vi "Lockin_sweep.vi"(0 "Transport":refnum<class "Transport.lvclass">, 3 "error in (no error)":errorcluster) -> (7 "Transport out":refnum<class "Transport.lvclass">, 10 "error out":errorcluster)   [LabVIEW 2019, in "Transport.lvclass"]
doc: "This VI uses the Lockin Sweep Method. That is, you tell the lockin to sweep from Start to End in a certain amount of time. The lockin will run independently while it executes the sweep. While the lockin is sweeping, this VI will poll the lockin once per second to get a snapshot of current results and the sweep status (sweeping or not sweeping). When the lockin is finished sweeping this VI will ask for the final sweep results and save them. The spacing between points is determined by the \"Fs Output\" control in the Lockin."
uses:
  Transport.lvclass
  <userlib>/LevyLab/Lockin-Multichannel/Instrument.DAQ/Typedefs/Sweep.Channel--Cluster--Array.ctl
  <userlib>/LevyLab/Lockin-Multichannel/Instrument.DAQ/Typedefs/Sweep.Channel--Cluster.ctl
  <userlib>/LevyLab/Lockin-Multichannel/Instrument.DAQ/Typedefs/Sweep.Pattern--Enum.ctl
  Transport.lvclass/Transport.ctl
  Control Experiment/Control Experiment.lvclass/Control Experiment.ctl
  Control Experiment/Typedefs/Instrument Types--enum.ctl
  <userlib>/LevyLab/Lockin-Multichannel/Instrument.Lockin/Typedefs/Results Type--Enum.ctl
  <userlib>/LevyLab/Lockin-Multichannel/Instrument.DAQ/Typedefs/Sweep.Configuration--Cluster.ctl
  <userlib>/LevyLab/Instrument Framework/Instrument Types/Cryostat/Typedefs/Magnet Axis--Enum.ctl
  Typedefs/Lockin_Sweep JSON--Cluster.ctl
  d7da78e6-7697-4005-8475-e4e7ed229128.vi
  <vilib>/PRIrvin/XY Utilities/subVIs/Multiply float (multiple).vi
  <vilib>/PRIrvin/XY Utilities/subVIs/Divide float (multiple).vi
  ac72d6f7-f5c3-431a-8621-5120436d0f52.vi
  217905a9-ad64-4e54-8703-31da4ffbd4c0.vi
  9896b5e5-a649-4b1b-acc0-fd49b17a1bc1.vi
  ac72d6f7-f5c3-431a-8621-5120436d0f52.vi/7eee748f-304e-47d8-aeea-bfc744331f26.vi
  ac72d6f7-f5c3-431a-8621-5120436d0f52.vi/d9440ba2-8dc0-48fa-8208-7fa22d71755a.vi
  <userlib>/LevyLab/Instrument Framework/Instrument/Instrument.lvclass
  C:/Program Files/National Instruments/LabVIEW 2019/vi.lib/JKI/JKI SMO/SMO/SMO.lvclass
  <userlib>/LevyLab/Instrument Framework/Instrument Types/Cryostat/Instrument.Cryostat.lvclass
  <userlib>/LevyLab/Lockin-Multichannel/Instrument.Lockin/Instrument.Lockin.lvclass
  C:/Program Files/National Instruments/LabVIEW 2019/user.lib/LevyLab/Instrument Framework/Instrument Types/Lockin/Instrument.LockinAPI.lvclass
  <userlib>/LevyLab/Debug/Debug/Get Debug Mode.vi
  <userlib>/LevyLab/Lockin-Multichannel/Instrument.Lockin/Private/Lockin.Remote Client.vi
  <vilib>/JDP Science/JSONtext/Variant to JSON Text.vi
  Control Experiment/subVIs/String Label.vi
  <vilib>/JKI/JKI SMO/SMO/SMO.lvclass
  Control Experiment/Control Experiment.lvclass
  <vilib>/JDP Science/JSONtext/LVClass Serializer/JSONtext LVClass Serializer.lvclass
  <userlib>/LevyLab/Instrument Framework/Instrument Types/CBridge/Instrument.CBridge.lvclass
  <userlib>/LevyLab/Instrument Framework/Instrument Types/Strain/Instrument.Strain.lvclass
  <userlib>/LevyLab/Instrument Framework/Instrument Types/Delay Line/Instrument.DelayLine.lvclass
  <userlib>/LevyLab/Lockin-Multichannel/Instrument.DAQ/Instrument.DAQ.lvclass
  <vilib>/PRIrvin/XY Utilities/xy_utilities.lvlib
  <vilib>/Utility/Data Type/NI_Data Type.lvlib
  <userlib>/LevyLab/Instrument Framework/Instrument Types/Lockin/Instrument.LockinAPI.lvclass
  <userlib>/LevyLab/Instrument Framework/Instrument Types/Amplifier/Instrument.Amplifier.lvclass
  <userlib>/LevyLab/Instrument Framework/Instrument Types/VNA/Instrument.VNA.lvclass
  <userlib>/LevyLab/Instrument Framework/Instrument Types/VSource/Instrument.VSource.lvclass
  Attributes/Instrument Attributes.lvlib
  <userlib>/LevyLab/Debug/Debug.lvlib
panel:
  in  "Start":bool
  in  "stop":bool
  out "Tab Control":T1(tab)
  in  "refresh (ms)":u32=1000
  out "state history":string
  in  "Sweep Tables":cluster{"Ch":i32, "Table":dbl[]}[](array[cluster]) {"Table" format="%#_3p"; "Ch" min=1 max=16}
  in  "Emergency Stop Visible?":bool
  out "elapsed time (s)":i32=231
  out "Experiment Comments":string
  out "Experiment Folder":string
  out "time b/w points (ms)":u32=1037
  in  "Sweep Channels":T2 {"Table" format="%#_1f"; "Channel" min=1 max=128; "Start" format="%#_6p"; "End" format="%#_6p"}
  in  "Sweep Time (s)":dbl
  in  "Initial Wait (s)":dbl
  in  "Return to Start":bool
  out "Instrument Status":string
  in  "Emergency Stop 1":bool caption="Emergency Stop"
  out "Lockin (X)":cluster{"Wavenumber":dbl[], "Data":dbl[]}[](graph)
  out "Lockin (Y)":cluster{"Wavenumber":dbl[], "Data":dbl[]}[](graph)
  in  "Units":enum16{"ohms & siemens", "h/e2 & e2/h"}(ring)
  out "Resistance":cluster{"X-array":dbl[], "Y-array":dbl[]}[](graph)
  out "Conductance":cluster{"X-array":dbl[], "Y-array":dbl[]}[](graph)
  in  "Emergency Stop 2":bool caption="Emergency Stop"
  out "AI":cluster{"Wavenumber":dbl[], "Data":dbl[]}[](graph)
  out "AO":cluster{"Wavenumber":dbl[], "Data":dbl[]}[](graph)
  in  "Emergency Stop 3":bool caption="Emergency Stop"
  out "2 Terminal":cluster{"Wavenumber":dbl[], "Data":dbl[]}[](graph)
  out "4 Terminal":cluster{"Wavenumber":dbl[], "Data":dbl[]}[](graph)
  in  "Emergency Stop 4":bool caption="Emergency Stop"
  # "Configuration"
  # "Status"
  # "Metadata*"
  # "VI Description"
  # "Run a sweep on the lockin itself. The lockin is told to sweep from Start to End over a set time, and it runs the sweep on its own. While it sweeps, this VI polls the lockin once per fresh time for a snapshot of the current results and the sweep status. When the sweep finishes, it reads the final sweep results and saves them. The point spacing is set by the lockin's \"Fs Output\" control."
  # "*Change these values in Transport Server"
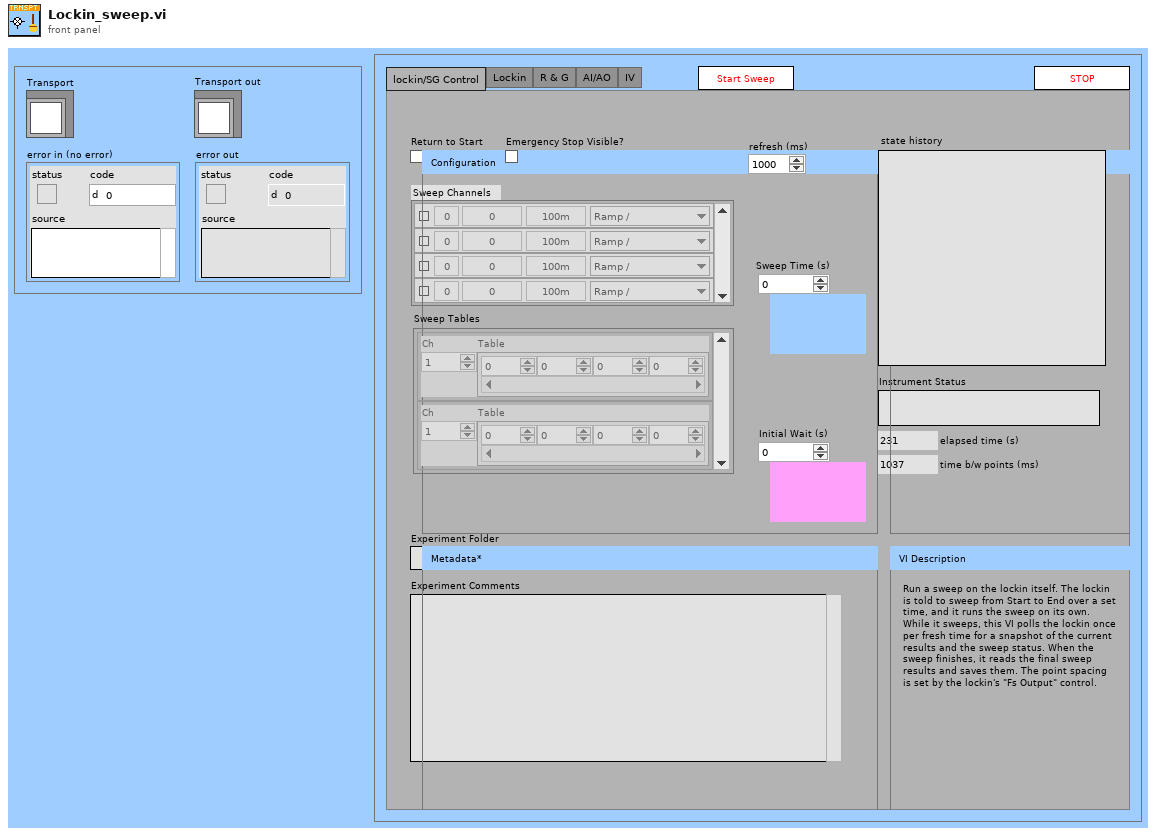
[diagram p1: front panel]
types:
  T1 = enum32{"lockin/SG Control", "Lockin", "R & G", "AI/AO", "IV"}
  T2 = typedef "Instrument.Lockin.lvlib/Instrument.DAQ.lvclass/Sweep.Channel--Cluster--Array.ctl" = T3[]
  T3 = typedef "Instrument.Lockin.lvlib/Instrument.DAQ.lvclass/Sweep.Channel--Cluster.ctl" = cluster{"Enable?":bool, "Channel":u16, "Start":dbl, "End":dbl, "Pattern":T4, "Table":dbl[]}
  T4 = typedef "Instrument.Lockin.lvlib/Instrument.DAQ.lvclass/Sweep.Pattern--Enum.ctl" = enum16{"Ramp /", "Ramp /\\", "Smooth Ramp _/", "Smooth Ramp _/\\_", "Table"}
  T5 = enum32{"Invalid", "Standard", "Closed", "Hidden", "Minimized", "Maximized"}
  T6 = enum32{"invalid app kind", "Development System", "Run Time System", "Student Edition", "Embedded LabVIEW", "Evaluation", "Custom"}
  T7 = enum32{"Bad", "Idle", "Run top level", "Running"}
  T8 = typedef "Control Experiment.lvclass/Instrument Types--enum.ctl" = enum16{"DAQ", "Amplifier", "Temperature", "Magnet", "Rotator", "Level", "Capacitance", "Delay Line", "Strain Cell", "VNA", "Source"}
  T9 = typedef "Instrument.Lockin.lvlib/Instrument.Lockin.lvclass/Results Type--Enum.ctl" = enum16{"X", "Y", "R", "Theta", "Mean"}
  T10 = typedef "Instrument.Lockin.lvlib/Instrument.DAQ.lvclass/Sweep.Configuration--Cluster.ctl" = cluster{"sweepTime":dbl, "initialWaitTime":dbl, "returnToStart":bool, "sweepChannels":T2}
  T11 = typedef "Instrument.Cryostat.lvclass/Magnet Axis--Enum.ctl" = enum16{"X", "Y", "Z"}
  T12 = typedef "Transport.lvclass/Lockin_Sweep JSON--Cluster.ctl" = cluster{"initialWaitTime":dbl, "sweepTime":dbl, "Return to Start":bool, "sweepChannels":T2, "sweepTables":cluster{"Ch":i32, "Table":dbl[]}[]}
  T13 = typedef "Control Experiment.lvclass/Instrument Classes--cluster.ctl" = cluster{"DAQ":refnum<class "Instrument.LockinAPI.lvclass">, "Amplifier":refnum<class "Instrument.Amplifier.lvclass">, "Temperature":refnum<class "Instrument.Cryostat.lvclass">, "Magnet":refnum<class "Instrument.Cryostat.lvclass">, "Rotator":refnum<class "Instrument.Cryostat.lvclass">, "Level":refnum<class "Instrument.Cryostat.lvclass">, "Capacitance":refnum<class "Instrument.CBridge.lvclass">, "Delay Line":refnum<class "Instrument.DelayLine.lvclass">, "Strain Cell":refnum<class "Instrument.Strain.lvclass">, "VNA":refnum<class "Instrument.VNA.lvclass">, "Source":refnum<class "Instrument.VSource.lvclass">}
  T14 = cluster{"Core":cluster{"Current VI Reference":refnum<vi>, "Close Panel on Exit?":bool}, "Transport":refnum<class "Transport.lvclass">, "C.E.":refnum<class "Control Experiment.lvclass">, "Instruments":T13, "Time":dbl, "Temperature":dbl, "Magnet":dbl, "Results (Dictionary)":cluster{"key":string, "value":dbl}[], "Sweep Value":dbl, "ms [0]":u32, "ms [i]":u32, "Execution:State":enum32{"Bad", "Idle", "Run top level", "Running"}, "Run Time System?":bool, "AO Waveforrm":waveform(dbl)[], "AI Waveform":waveform(dbl)[], "Sweep_AO":waveform(dbl)[], "Sweep_AI":waveform(dbl)[], "Sweep_X":waveform(dbl)[], "Sweep_Y":waveform(dbl)[], "Amplitude":dbl[], "UI stop":bool}
  T15 = cluster{"Current VI Reference":refnum<vi>, "Close Panel on Exit?":bool}
  T16 = cluster{"I-":i32, "I+":i32, "V1-":i32, "V1+":i32, "I2-":i32, "I2+":i32, "V2-":i32, "V2+":i32}
  T17 = typedef "Instrument.LockinAPI.lvclass/LockinAPI.getState.states--enum.ctl" = enum16{"idle", "created", "started", "stopped", "sweeping"}
  T18 = typedef "Instrument.Lockin.lvlib/Instrument.DAQ.lvclass/AO.Channel--Cluster--Array.ctl" = T19[]
  T19 = typedef "Instrument.Lockin.lvlib/Instrument.DAQ.lvclass/AO.Channel--Cluster.ctl" = cluster{"Enable?":bool, "Channel":i32, "Amplitude":dbl, "Offset":dbl, "Frequency":dbl, "Phase":dbl, "Function":T20, "Sweeping?":bool, "Limit AC":bool, "Limit DC?":bool, "Duty Cycle":bool}
  T20 = typedef "Instrument.Lockin.lvlib/Instrument.DAQ.lvclass/AO.Channel.Function--Enum.ctl" = enum16{"sine", "square", "triangle", "saw"}
  T21 = typedef "Instrument.LockinAPI.lvclass/LockinAPI.SweepData--Cluster.ctl" = cluster{"AO":waveform(dbl)[], "AI":waveform(dbl)[], "X":waveform(dbl)[], "Y":waveform(dbl)[]}
  T22 = typedef "LV-Data.lvclass/Dictionary--cluster.ctl" = cluster{"key":string, "value":variant}
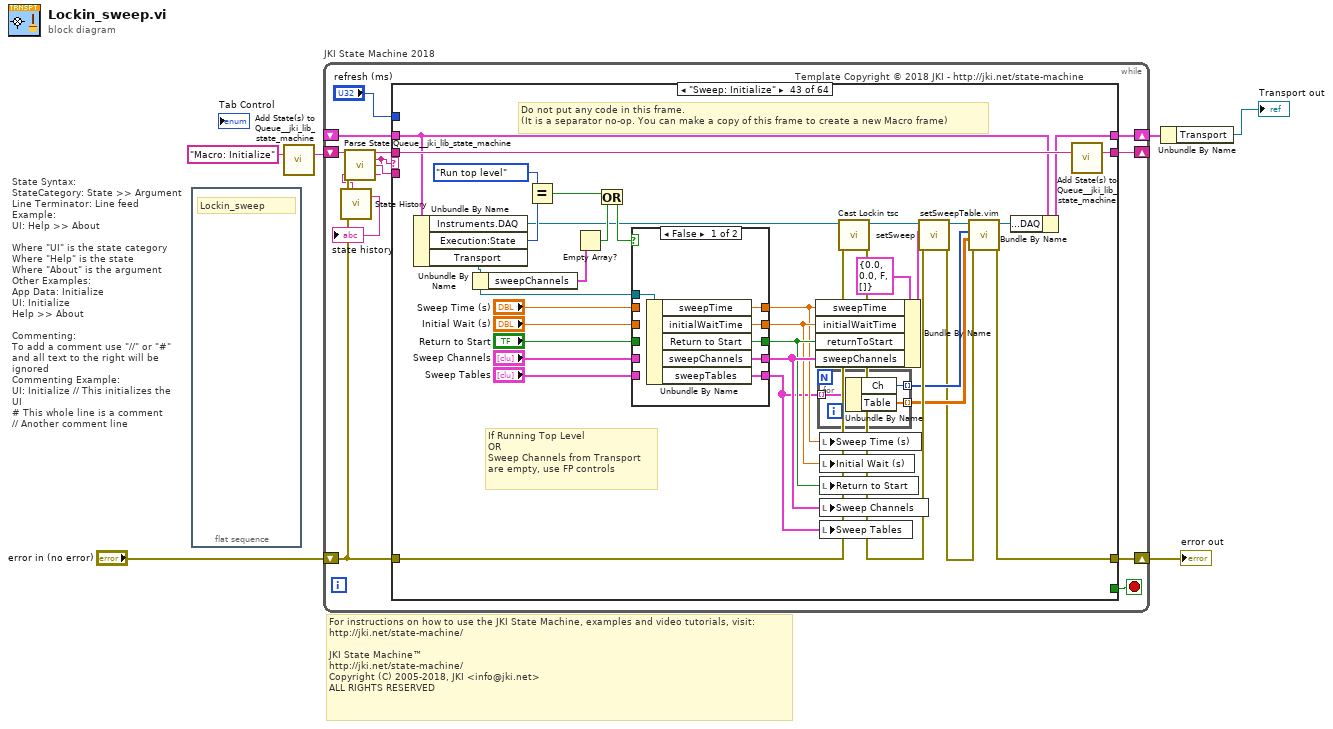
[diagram p0: block diagram]
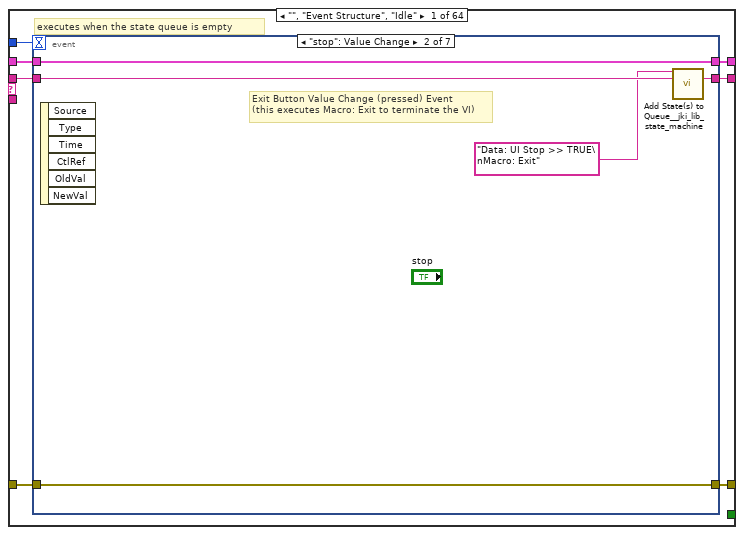
[diagram p2: hidden frame]
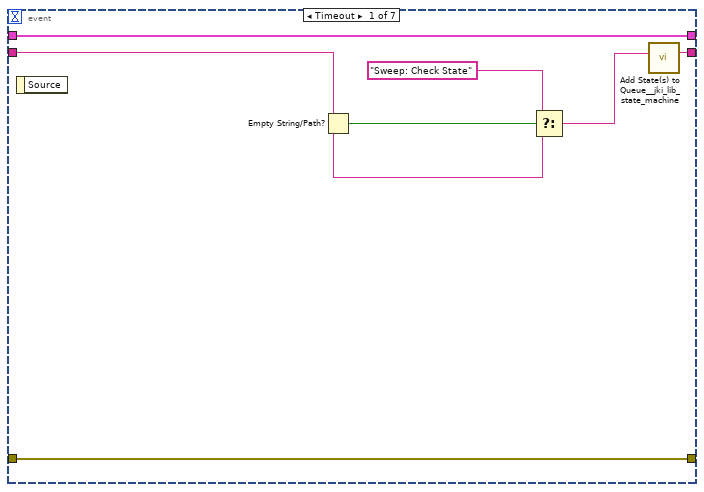
[diagram p3: hidden frame]
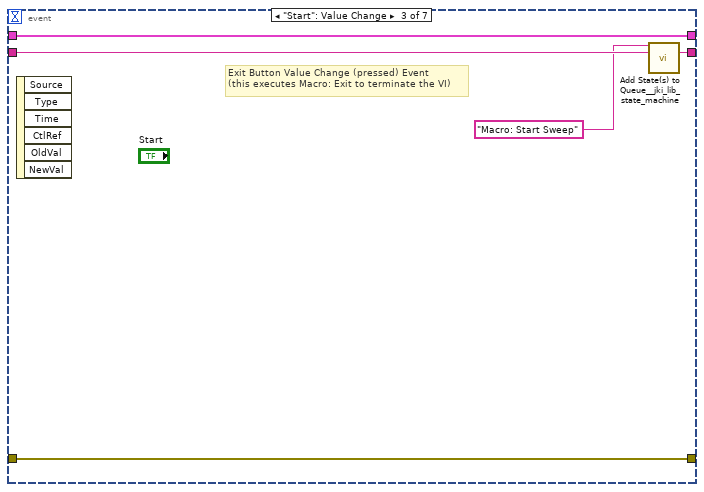
[diagram p4: hidden frame]
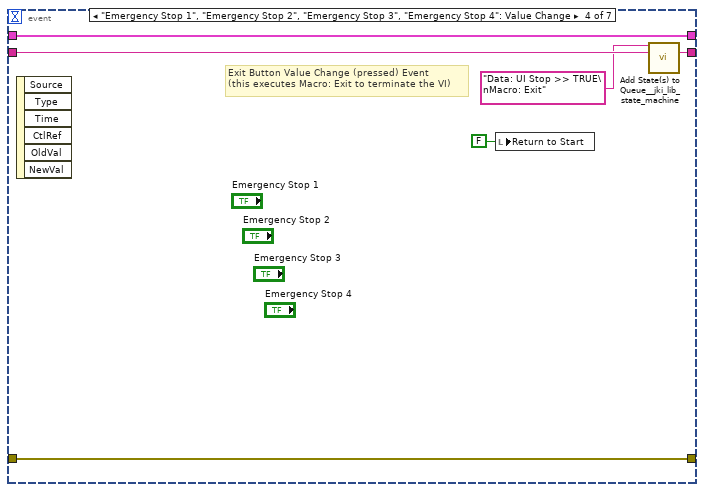
[diagram p5: hidden frame]
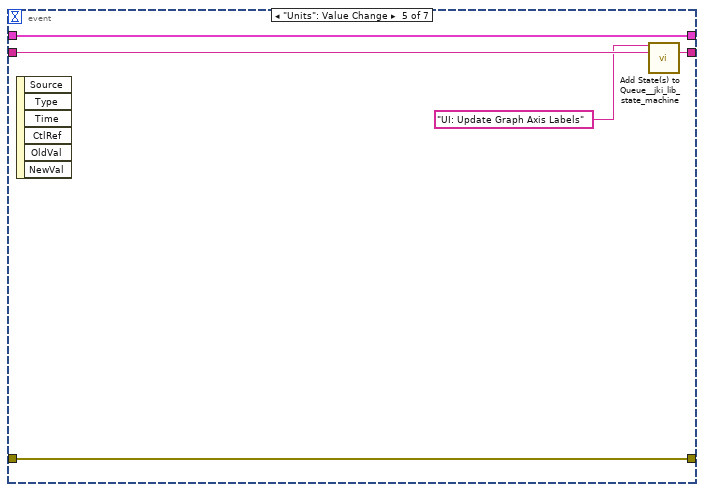
[diagram p6: hidden frame]
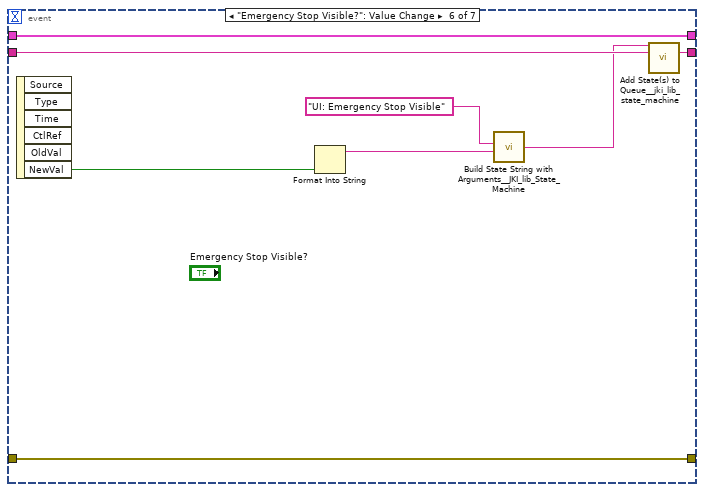
[diagram p7: hidden frame]
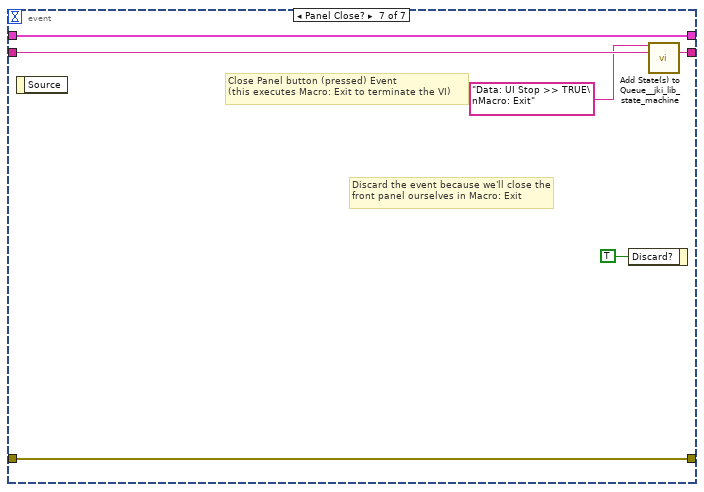
[diagram p8: hidden frame]
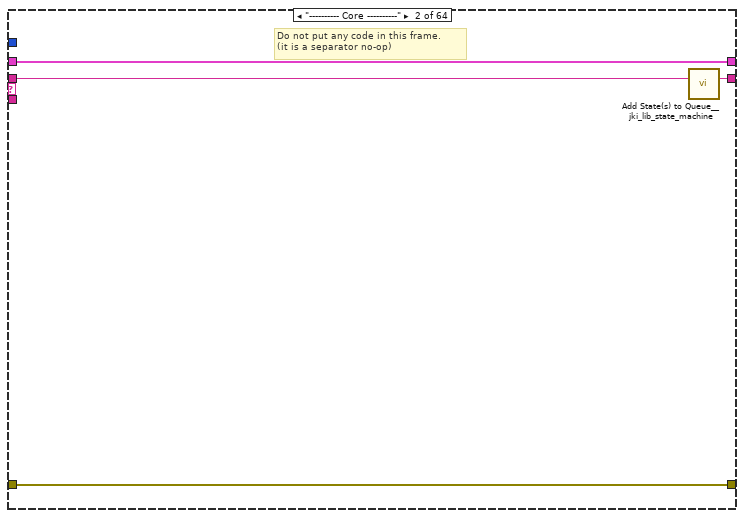
[diagram p9: hidden frame]
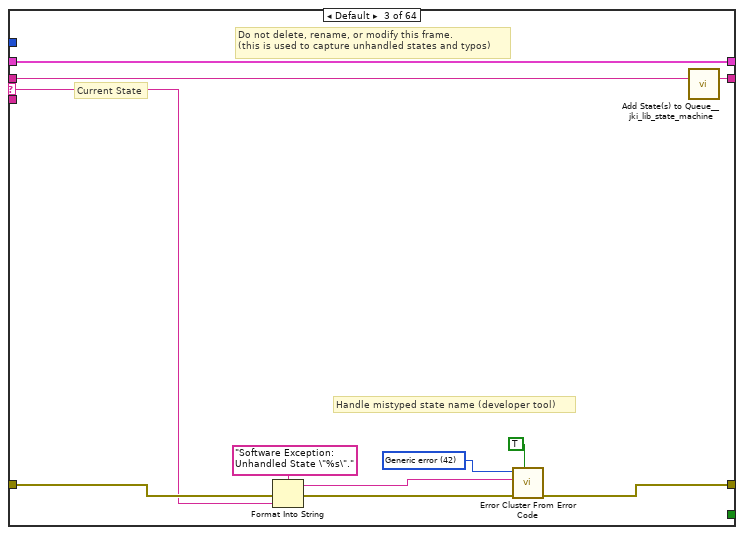
[diagram p10: hidden frame]
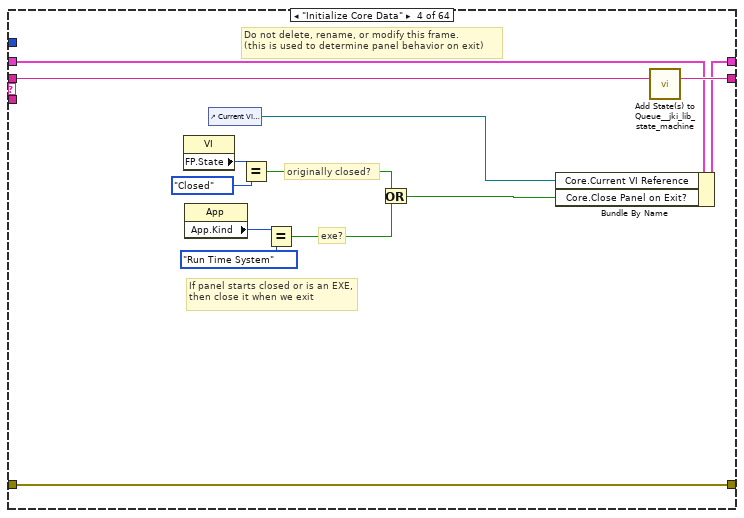
[diagram p11: hidden frame]
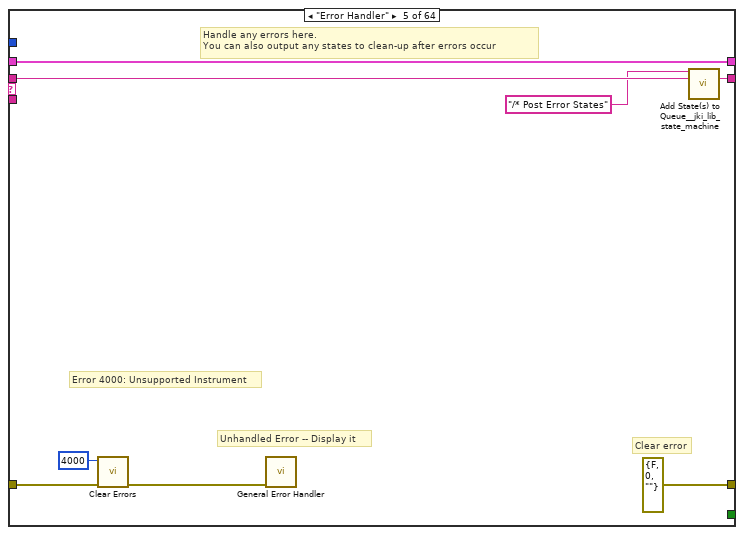
[diagram p12: hidden frame]
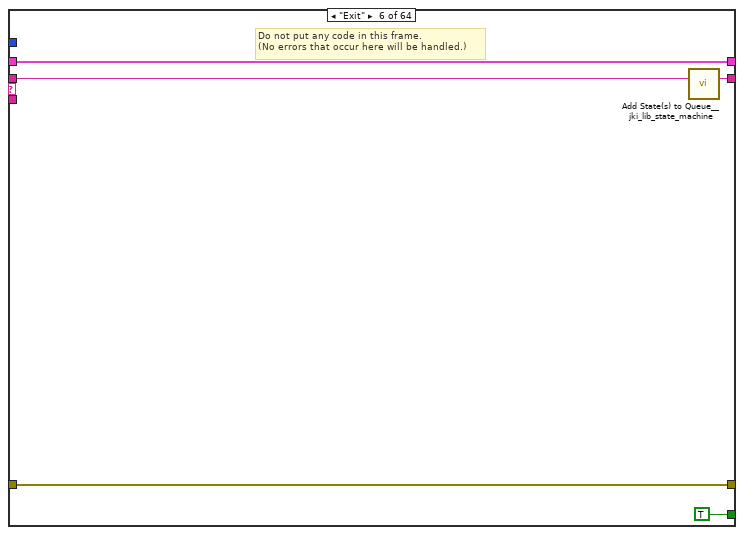
[diagram p13: hidden frame]
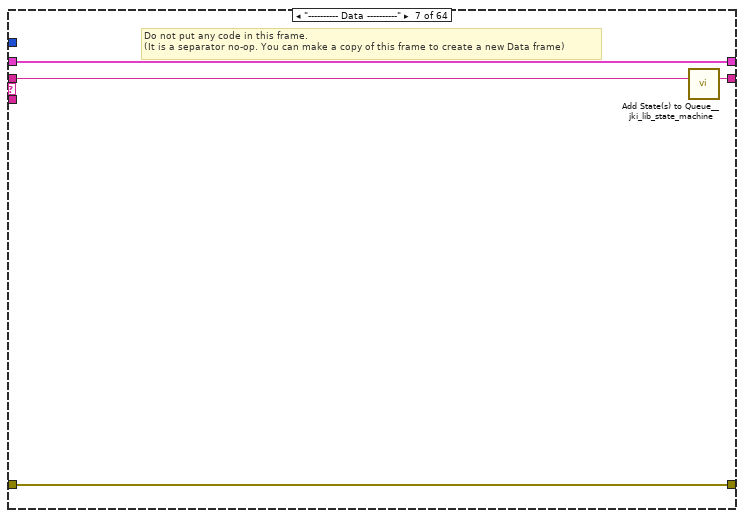
[diagram p14: hidden frame]
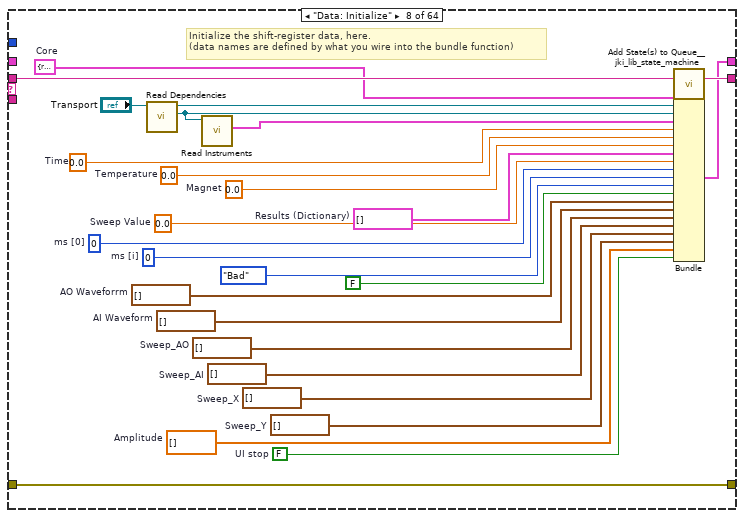
[diagram p15: hidden frame]
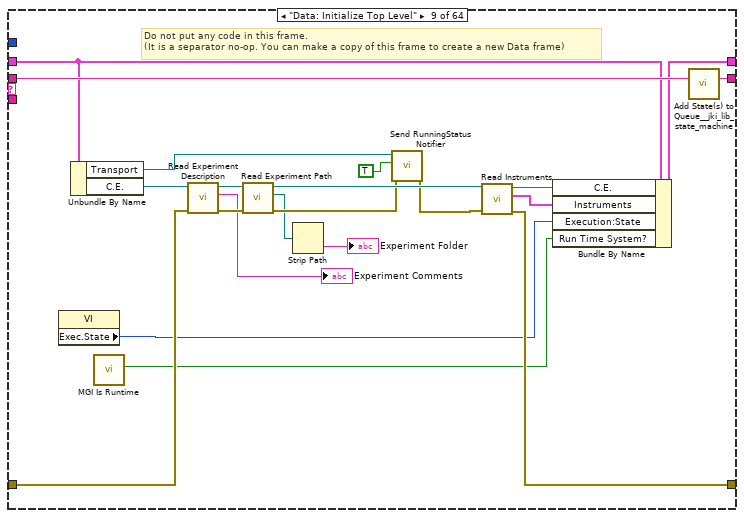
[diagram p16: hidden frame]
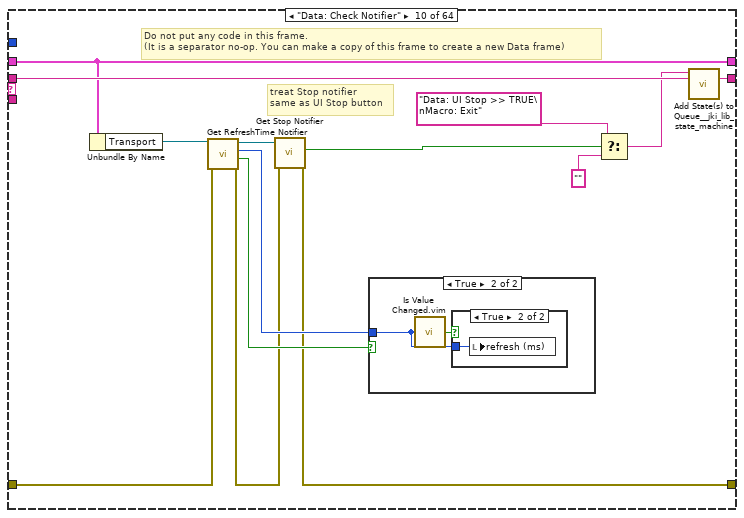
[diagram p17: hidden frame]
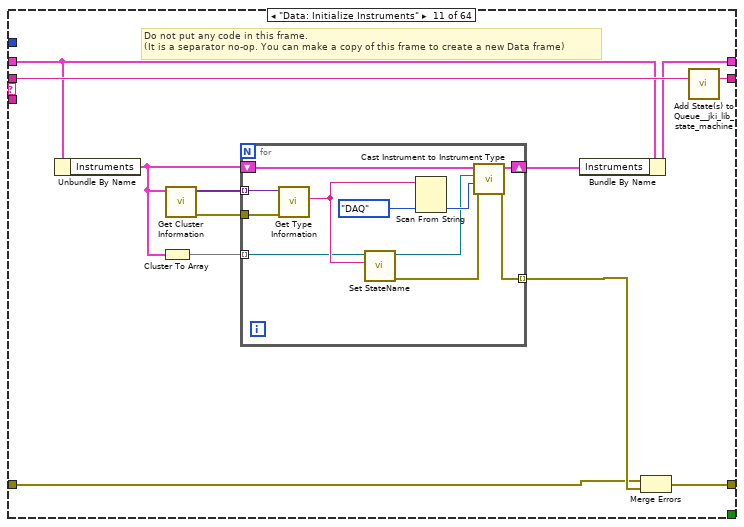
[diagram p20: hidden frame]
diagram:
  # "For instructions on how to use the JKI State Machine, examples and video tutorials, visit:\nhttp://jki.net/state-machine/\n\nJKI State Machine™\nhttp://jki.net/state-machine/\nCopyright (C) 2005-2018, JKI <info@jki.net>\nALL RIGHTS RESERVED"
  # "State Syntax:\nStateCategory: State >> Argument\nLine Terminator: Line feed\nExample:\nUI: Help >> About\n\nWhere \"UI\" is the state category\nWhere \"Help\" is the state\nWhere \"About\" is the argument\nOther Examples:\nApp Data: Initialize\nUI: Initialize\nHelp >> About\n\nCommenting:\nTo add a comment use \"//\" or \"#\" and all text to the right will be ignored\nCommenting Example:\nUI: Initialize // This initializes the UI\n# This whole line is a comment\n// Another comment line"
  n1 = flat-sequence {
    frame #0 {
      # "Lockin_sweep"
    }
  }
  n2 = call <vilib>:"Add State(s) to Queue__jki_lib_state_machine.vi"("State(s) in (\"\")"="Macro: Initialize") -> ("States Out"=w6:string)  [unwired: 14 in]
  n3 = while "JKI State Machine 2018" {
    shift-right: [w13] -> w4
    shift-left: _ -> [w12]
    shift-right: [w16] -> w2
    shift-left: "error in (no error)" -> [w11]
    shift-right: [w15] -> _
    shift-left: w6 -> [w10]
    stop <- w14 stop-if-true
    # "Template Copyright © 2018 JKI - http://jki.net/state-machine"
    n4 = call <vilib>:"Parse State Queue__jki_lib_state_machine.vi"("State Queue"=w10, "Error In (no error)"=w11) -> ("Remaining States"=w18:string, "Current State"=w9:string, "Arguments"=w17:string)  [unwired: 11 in]
    n5 = call <userlib>:"State History.vi"("Current State"=w9) -> ("History"=→"state history":string)  [unwired: 9 in, 1 out]
    n6 = case shown="\"Sweep: Initialize\"" w9 {
      selector: w9 -> [_ _ w72 _ _ _ _ _ _ _ _ _ _ _ _ _ _ _ _ _ _ _ _ _ _ _ _ _ _ _ _ _ _ _ _ _ _ _ _ _ _ _ _ _ _ _ _ _ _ _ _ _ _ _ _ _ _ _ _ _ _ _ _ _]
      tunnel: w18 -> [w25 w71 w76 w95 w103 w108 w112 w138 w159 w173 w188 w212 w243 w278 w290 w317 w338 w350 w361 w367 w378 w394 w409 w435 w452 w472 w510 w559 w584 w599 w617 w664 w676 w745 w755 w760 w773 w786 w791 w803 w814 w818 w851 w877 w889 w903 w927 w940 w944 w948 w959 w974 w996 w1024 w1057 w1079 w1101 w1123 w1155 w1176 w1180 w1184 w1204 w1223]
      tunnel: w17 -> [_ _ _ _ _ _ _ _ _ _ _ _ _ _ _ w312 _ _ _ w362 w374 _ w396 _ _ _ _ w553 w573 _ _ _ w670 _ _ _ _ _ _ _ _ _ _ _ _ _ _ _ _ _ _ _ _ _ _ _ _ _ _ _ _ _ _ _]
      tunnel: w12 -> [w23 w68 w74 w88 w100 w106 w109 _ w149 w164 w185 w209 w240 w263 w284 w313 w332 w347 w352 w365 w375 w390 w406 w425 w448 w469 w507 w557 w576 w591 w614 w654 w672 w742 w748 w757 w769 w782 w787 w795 w811 w815 w848 w875 w883 w901 w925 w937 w942 w945 w952 w968 w989 w1015 w1051 w1073 w1095 w1117 w1147 w1174 w1177 w1181 w1192 w1218]
      tunnel: [w22 w69 w78 w92 errorcluster {"status"=FALSE, "code"=0, "source"=""} ("error out") w105 w110 w135 w151 w162 w184 w202 w239 w265 w282 w315 w333 w348 w354 w363 w376 w386 w407 w430 w450 w470 w508 w556 w577 w597 w615 w645 w673 w743 w753 w758 w762 w784 w789 w801 w812 w816 w819 w870 w887 w896 w914 w938 w941 w946 w950 w962 w984 w1013 w1044 w1067 w1089 w1111 w1153 w1171 w1178 w1182 w1195 w1216] -> w16
      tunnel: w11 -> [w21 w69 w77 w92 w97 w105 w110 w135 w152 w161 w177 w203 w238 w272 w285 w315 w324 w348 w359 w364 w376 w381 w407 w429 w446 w461 w494 w556 w571 w597 w615 w646 w674 w743 w753 w758 w761 w784 w789 w801 w812 w816 w825 w866 w878 w892 w904 w938 w941 w946 w951 w972 w991 w1011 w1052 w1074 w1096 w1118 w1131 w1162 w1178 w1182 w1187 w1211]
      tunnel: [w24 w70 w75 w94 w102 w107 w111 w137 w158 w172 w187 w211 w242 w277 w289 w316 w337 w349 w360 w366 w377 w393 w408 w434 w451 w471 w509 w558 w583 w598 w616 w663 w675 w744 w754 w759 w772 w785 w790 w802 w813 w817 w850 w876 w888 w902 w926 w939 w943 w947 w958 w973 w995 w1023 w1056 w1078 w1100 w1122 w1154 w1175 w1179 w1183 w1203 w1222] -> w15
      tunnel: [_ _ _ _ _ TRUE _ _ _ _ _ _ _ _ _ _ _ _ _ _ _ _ _ _ _ _ _ _ _ _ _ _ _ _ _ _ _ _ _ _ _ _ _ _ _ _ _ _ _ _ _ _ _ _ _ _ _ _ _ _ _ _ _ _] -> w14
      tunnel: [w20 w68 w74 w93 w100 w106 w109 w136 w150 w164 w186 w210 w241 w273 w283 w314 w335 w347 w355 w365 w375 w389 w406 w425 w448 w469 w507 w557 w576 w591 w614 w654 w672 w742 w748 w757 w769 w782 w787 w795 w811 w815 w849 w874 w884 w900 w924 w937 w942 w945 w956 w971 w994 w1016 w1055 w1077 w1099 w1121 w1146 w1173 w1177 w1181 w1193 w1219] -> w13
      tunnel: "refresh (ms)" -> [w19 _ _ _ _ _ _ _ _ _ _ _ _ _ _ _ _ _ _ _ _ _ _ _ _ _ _ _ _ _ _ _ _ _ _ _ _ _ _ _ _ _ _ _ _ _ _ _ _ _ _ _ _ _ _ _ _ _ _ _ _ _ _ _]
      frame "", "Event Structure", "Idle" {
        # "executes when the state queue is empty"
        n7 = event shown="[1] \"stop\": Value Change" {
          selector: _ -> [_ _ _ _ _ _ _]
          dyn-events: _ -> [_ _ _ _ _ _ _]
          timeout: w19 -> [_ _ _ _ _ _ _]
          tunnel: w25 -> [w27 w37 w42 w48 w53 w61 w67]
          tunnel: [w32 w36 w41 w47 w52 w60 w66] -> w24
          tunnel: w23 -> [w30 w33 w38 w45 w50 w58 w64]
          tunnel: [w31 w35 w40 w46 w51 w59 w65] -> w22
          tunnel: w21 -> [w31 w35 w40 w46 w51 w59 w65]
          tunnel: [w30 w33 w38 w45 w50 w58 w64] -> w20
          event Timeout {
            n8 = event-data() -> ()  [unwired: 1 in, 1 out]
            n9 = Empty String/Path?(string/path=w27) -> (empty?=w29:bool)
            n10 = Select(t="Sweep: Check State" ("State(s) in Front (\"\")"), s=w29, f=w27) -> (s? t:f=w28:string)
            n11 = call <vilib>:"Add State(s) to Queue__jki_lib_state_machine.vi"("State(s) in (\"\")"=w28) -> ("States Out"=w32:string)  [unwired: 14 in]
          }
          event "stop": Value Change {
            # "Exit Button Value Change (pressed) Event\n(this executes Macro: Exit to terminate the VI)"
            n12 = event-data() -> ()  [unwired: 1 in, 6 out]
            n13 = call <vilib>:"Add State(s) to Queue__jki_lib_state_machine.vi"("State(s) in Front (\"\")"="Data: UI Stop >> TRUE\nMacro: Exit", "State(s) in (\"\")"=w37) -> ("States Out"=w36:string)  [unwired: 13 in]
          }
          event "Start": Value Change {
            # "Exit Button Value Change (pressed) Event\n(this executes Macro: Exit to terminate the VI)"
            n14 = event-data() -> ()  [unwired: 1 in, 6 out]
            n15 = call <vilib>:"Add State(s) to Queue__jki_lib_state_machine.vi"("State(s) in Front (\"\")"="Macro: Start Sweep", "State(s) in (\"\")"=w42) -> ("States Out"=w41:string)  [unwired: 13 in]
          }
          event "Emergency Stop 1", "Emergency Stop 2", "Emergency Stop 3", "Emergency Stop 4": Value Change {
            # "Exit Button Value Change (pressed) Event\n(this executes Macro: Exit to terminate the VI)"
            n16 = event-data() -> ()  [unwired: 1 in, 6 out]
            n17 = local write "Return to Start"(FALSE ("Return to Start")) -> ()
            n18 = call <vilib>:"Add State(s) to Queue__jki_lib_state_machine.vi"("State(s) in Front (\"\")"="Data: UI Stop >> TRUE\nMacro: Exit", "State(s) in (\"\")"=w48) -> ("States Out"=w47:string)  [unwired: 13 in]
          }
          event "Units": Value Change {
            n19 = event-data() -> ()  [unwired: 1 in, 6 out]
            n20 = call <vilib>:"Add State(s) to Queue__jki_lib_state_machine.vi"("State(s) in Front (\"\")"="UI: Update Graph Axis Labels", "State(s) in (\"\")"=w53) -> ("States Out"=w52:string)  [unwired: 13 in]
          }
          event "Emergency Stop Visible?": Value Change {
            n21 = event-data() -> ("NewVal"=w55:bool)  [unwired: 1 in, 5 out]
            n22 = Format Into String(w55) -> (resulting string=w57:string)  [unwired: 3 in, 1 out]
            n23 = call <vilib>:"Build State String with Arguments__JKI_lib_State_Machine.vi"("Arguments (\"\")"=w57, "State"="UI: Emergency Stop Visible") -> ("State with Arguments"=w54:string)  [unwired: 4 in]
            n24 = call <vilib>:"Add State(s) to Queue__jki_lib_state_machine.vi"("State(s) in Front (\"\")"=w54, "State(s) in (\"\")"=w61) -> ("States Out"=w60:string)  [unwired: 13 in]
          }
          event Panel Close? {
            # "Discard the event because we'll close the front panel ourselves in Macro: Exit"
            # "Close Panel button (pressed) Event\n(this executes Macro: Exit to terminate the VI)"
            n25 = event-data() -> ()  [unwired: 1 in, 1 out]
            n26 = event-data("Discard?"=TRUE) -> ()  [unwired: 1 in, 1 out]
            n27 = call <vilib>:"Add State(s) to Queue__jki_lib_state_machine.vi"("State(s) in Front (\"\")"="Data: UI Stop >> TRUE\nMacro: Exit", "State(s) in (\"\")"=w67) -> ("States Out"=w66:string)  [unwired: 13 in]
          }
        }
      }
      frame "---------- Core ----------" {
        # "Do not put any code in this frame.\n(it is a separator no-op)"
        n28 = call <vilib>:"Add State(s) to Queue__jki_lib_state_machine.vi"("State(s) in (\"\")"=w71) -> ("States Out"=w70:string)  [unwired: 14 in]
      }
      frame Default {
        w81 = 42 items=["No error", "Argument error", "Memory is full", "Out of zone", "End of file", "File already open", "Generic file I/O error", "File not found", "File permission error", "Disk is full", "Duplicate path", "Too many files open", "System feature not enabled", "Resource file not found", "Cannot add resource", "Resource not found", "Image not found", "Image memory error", "Pen does not exist", "Config type invalid", "Config token not found", "Config parse error", "Config memory error", "Bad external code format", "Bad external code offset", "External code not present", "Null window", "Destroy window error", "Null menu", "Print aborted", "Bad print record", "Print driver error", "Windows error during printing", "Memory error during printing", "Print dialog error", "Generic print error", "Invalid device refnum", "Device not found", "Device parameter error", "Device unit error", "Cannot open device", "Device call aborted", "Generic error", "Cancelled by user", "Object ID too low", "Object ID too high", "Object not in heap", "Unknown heap", "Unknown object (invalid DefProc)", "Unknown object (DefProc not in table)", "Message out of range", "Invalid (null) method", "Unknown message", "Manager call not supported", "Bad address", "Network operation in progress", "Network operation timed out", "Connection is busy", "Network attribute not supported", "Network error", "Address in use", "System out of memory", "Connection aborted", "Connection refused", "Not connected", "Already connected", "Connection closed", "Initialization error (interapplication manager)", "Bad occurrence", "Wait on unbound occurrence handler", "Occurrence queue overflow", "Datalog type conflict", "Unused", "Unrecognized type (interapplication manager)", "Memory corrupt", "Failed to make temporary DLL", "Old CIN version", "Drag socket not found", "Failed to load drop-object", "Failed to register OLE object", "Failed to release OLE object", "Format specifier type mismatch", "Unknown format specifier", "Too few format specifiers", "Too many format specifiers", "Scan failed", "Newer CIN version", "Error converting to variant", "Runtime menu error", "Password tampered", "Variant attribute not found", "Incompatible variant data type", "Event data is not available", "Event Store is not present", "Occurrence is not found", "Event Queue is not created", "Event info is not available", "Refnum passed is NULL", "Error retrieving Class GUID", "Error retrieving CoClass GUID", "Error retrieving TypeLib GUID.", "Bad built application magic bytes.", "Specific driver is different from the specific driver associated with the Logical Name.", "There is no session opened to the class driver.", "Max Error", "MAX - Error with config objects", "MAX - Error loading configuration", "MAX - Group not supported"]
        # "Current State"
        # "Do not delete, rename, or modify this frame.\n(this is used to capture unhandled states and typos)"
        # "Handle mistyped state name (developer tool)"
        n29 = Format Into String(format string="Software Exception: Unhandled State \"%s\"." ("message"), error in=w77, w72) -> (resulting string=w80:string, error out=w79:errorcluster)  [unwired: 1 in]
        n30 = call <vilib>:"Error Cluster From Error Code.vi"("show call chain? (False)"=TRUE, "error in (no error)"=w79, "error message (\"\")"=w80, "error code (0)"=w81) -> ("error out"=w78:errorcluster)  [unwired: 5 in]
        n31 = call <vilib>:"Add State(s) to Queue__jki_lib_state_machine.vi"("State(s) in (\"\")"=w76) -> ("States Out"=w75:string)  [unwired: 14 in]
      }
      frame "Initialize Core Data" {
        # "Do not delete, rename, or modify this frame.\n(this is used to determine panel behavior on exit)"
        # "originally closed?"
        # "exe?"
        # "If panel starts closed or is an EXE, then close it when we exit"
        n32 = property class="VI"() -> ("FP.State"=w85:T5)  [unwired: 2 in, 2 out]
        n33 = property class="App"() -> ("App.Kind"=w91:T6)  [unwired: 2 in, 2 out]
        n34 = control-ref of="Current VI Reference"() -> (w86:refnum<vi>)
        n35 = Equal?(x=w85, y=T5."Closed" ("Front Panel Window:State")) -> (x = y?=w83:bool)
        n36 = Equal?(x=w91, y=T6."Run Time System" ("Application:Kind")) -> (x = y?=w89:bool)
        n37 = Or(x=w83, y=w89) -> (x .or. y?=w87:bool)
        n38 = Bundle By Name(cluster=w88, "Core.Current VI Reference"=w86, "Core.Close Panel on Exit?"=w87) -> (w93:T14)
        n39 = call <vilib>:"Add State(s) to Queue__jki_lib_state_machine.vi"("State(s) in (\"\")"=w95) -> ("States Out"=w94:string)  [unwired: 14 in]
      }
      frame "Error Handler" {
        # "Error 4000: Unsupported Instrument"
        # "Unhandled Error -- Display it"
        # "Handle any errors here.\nYou can also output any states to clean-up after errors occur"
        # "Clear error"
        n40 = call <vilib>:"Clear Errors.vi"("error in (no error)"=w97, "specific error code to clear (0: all)"=4000) -> ("error out"=w96:errorcluster)  [unwired: 4 in, 1 out]
        n41 = call <vilib>:"General Error Handler.vi"("error in (no error)"=w96) -> ()  [unwired: 10 in, 5 out]
        n42 = call <vilib>:"Add State(s) to Queue__jki_lib_state_machine.vi"("State(s) in Front (\"\")"="/* Post Error States", "State(s) in (\"\")"=w103) -> ("States Out"=w102:string)  [unwired: 13 in]
      }
      frame "Exit" {
        # "Do not put any code in this frame.\n(No errors that occur here will be handled.)"
        n43 = call <vilib>:"Add State(s) to Queue__jki_lib_state_machine.vi"("State(s) in (\"\")"=w108) -> ("States Out"=w107:string)  [unwired: 14 in]
      }
      frame "---------- Data ----------" {
        # "Do not put any code in this frame.\n(It is a separator no-op. You can make a copy of this frame to create a new Data frame)"
        n44 = call <vilib>:"Add State(s) to Queue__jki_lib_state_machine.vi"("State(s) in (\"\")"=w112) -> ("States Out"=w111:string)  [unwired: 14 in]
      }
      frame "Data: Initialize" {
        w115 = FALSE  # UI stop
        w118 = dbl[] []  # Amplitude
        w122 = waveform(dbl)[] []  # Sweep_Y
        w123 = waveform(dbl)[] []  # Sweep_X
        w119 = cluster{"key":string, "value":dbl}[] []  # Results (Dictionary)
        w125 = waveform(dbl)[] []  # Sweep_AO
        w124 = waveform(dbl)[] []  # Sweep_AI
        w126 = waveform(dbl)[] []  # AI Waveform
        w127 = waveform(dbl)[] []  # AO Waveforrm
        w128 = 0.0  # Sweep Value
        w129 = u32 0  # ms [i]
        w130 = u32 0  # ms [0]
        w132 = 0.0  # Time
        w133 = 0.0  # Magnet
        w131 = 0.0  # Temperature
        w134 = T15 {"Current VI Reference"=refnum, "Close Panel on Exit?"=FALSE}  # Core
        # "Initialize the shift-register data, here.\n(data names are defined by what you wire into the bundle function)"
        n45 = call "Read Dependencies.vi"("Transport"="Transport") -> ("C.E."=w117:refnum<class "Control Experiment.lvclass">, "Transport"=w120:refnum<class "Transport.lvclass">)  [unwired: 8 in, 1 out]
        n46 = call "Read Instruments.vi"("Control Experiment in"=w117) -> ("Instruments"=w116:T13)  [unwired: 8 in, 2 out]
        n47 = call <vilib>:"Add State(s) to Queue__jki_lib_state_machine.vi"("State(s) in (\"\")"=w138) -> ("States Out"=w137:string)  [unwired: 14 in]
        n48 = Bundle("Core"=w134, "Transport"=w120, "C.E."=w117, "Instruments"=w116, "Time"=w132, "Temperature"=w131, "Magnet"=w133, "Results (Dictionary)"=w119, "Sweep Value"=w128, "ms [0]"=w130, "ms [i]"=w129, "Execution:State"=T7."Bad", "Run Time System?"=FALSE, "AO Waveforrm"=w127, "AI Waveform"=w126, "Sweep_AO"=w125, "Sweep_AI"=w124, "Sweep_X"=w123, "Sweep_Y"=w122, "Amplitude"=w118, "UI stop"=w115) -> (w136:T14)  [unwired: 1 in]
      }
      frame "Data: Initialize Top Level" {
        # "Do not put any code in this frame.\n(It is a separator no-op. You can make a copy of this frame to create a new Data frame)"
        n49 = property class="VI"() -> ("Exec.State"=w148:T7)  [unwired: 2 in, 2 out]
        n50 = Unbundle By Name(w149) -> ("Transport"=w146:refnum<class "Transport.lvclass">, "C.E."=w153:refnum<class "Control Experiment.lvclass">)
        n51 = call <userlib>:"MGI Is Runtime.vi"() -> ("Run Time System?"=w147:bool)  [unwired: 7 in]
        n52 = call "Read Experiment Description.vi"("error in (no error)"=w152, "Control Experiment in"=w153) -> ("error out"=w145:errorcluster, "Experiment Description"=→"Experiment Comments":string, "Control Experiment out"=w144:refnum<class "Control Experiment.lvclass">)  [unwired: 7 in]
        n53 = call "Read Experiment Path.vi"("error in (no error)"=w145, "Control Experiment in"=w144) -> ("error out"=w142:errorcluster, "Experiment Path"=w139:path, "Control Experiment out"=w155:refnum<class "Control Experiment.lvclass">)  [unwired: 7 in]
        n54 = Strip Path(path=w139) -> (name=→"Experiment Folder":string)  [unwired: 1 out]
        n55 = call "Send RunningStatus Notifier.vi"("error in (no error)"=w142, "Running?"=TRUE, "Transport in"=w146) -> ("error out"=w154:errorcluster)  [unwired: 7 in, 1 out]
        n56 = call "Read Instruments.vi"("error in (no error)"=w154, "Control Experiment in"=w155) -> ("error out"=w151:errorcluster, "Instruments"=w157:T13, "Control Experiment out"=w156:refnum<class "Control Experiment.lvclass">)  [unwired: 7 in]
        n57 = Bundle By Name(cluster=w149, "C.E."=w156, "Instruments"=w157, "Execution:State"=w148, "Run Time System?"=w147) -> (w150:T14)
        n58 = call <vilib>:"Add State(s) to Queue__jki_lib_state_machine.vi"("State(s) in (\"\")"=w159) -> ("States Out"=w158:string)  [unwired: 14 in]
      }
      frame "Data: Check Notifier" {
        # "treat Stop notifier\nsame as UI Stop button"
        # "Do not put any code in this frame.\n(It is a separator no-op. You can make a copy of this frame to create a new Data frame)"
        n59 = Unbundle By Name(w164) -> ("Transport"=w168:refnum<class "Transport.lvclass">)
        n60 = call "Get RefreshTime Notifier.vi"("error in (no error)"=w161, "Transport in"=w168) -> ("error out"=w163:errorcluster, "valid?"=w165:bool, "RefreshTime (ms)"=w166:u32, "Transport out"=w167:refnum<class "Transport.lvclass">)  [unwired: 6 in]
        n61 = call "Get Stop Notifier.vi"("error in (no error)"=w163, "Transport in"=w167) -> ("error out"=w162:errorcluster, "Stop?"=w160:bool)  [unwired: 7 in, 1 out]
        n62 = case shown="True" w165 {
          tunnel: w166 -> [_ w174]
          frame False {
          }
          frame True {
            n63 = call "Is Value Changed.vim"("value"=w174) -> ("changed or first call?"=w175:bool)
            n64 = case shown="True" w175 {
              tunnel: w174 -> [_ w176]
              frame False {
              }
              frame True {
                n65 = local write "refresh (ms)"(w176) -> ()
              }
            }
          }
        }
        n66 = Select(t="Data: UI Stop >> TRUE\nMacro: Exit", s=w160, f="") -> (s? t:f=w169:string)
        n67 = call <vilib>:"Add State(s) to Queue__jki_lib_state_machine.vi"("State(s) in Front (\"\")"=w169, "State(s) in (\"\")"=w173) -> ("States Out"=w172:string)  [unwired: 13 in]
      }
      frame "Data: Initialize Instruments" {
        # "Do not put any code in this frame.\n(It is a separator no-op. You can make a copy of this frame to create a new Data frame)"
        n68 = Unbundle By Name(w185) -> ("Instruments"=w178:T13)
        n69 = Cluster To Array(cluster=w178) -> (array=w183:refnum<class "Instrument.lvclass">[])
        n70 = call <vilib>:"Get Cluster Information.vi"("variant"=w178) -> ("error out"=w181:errorcluster, "cluster elements"=w182:variant[])  [unwired: 9 in]
        n71 = for {
          tunnel: w183 -> [w189] mode=indexing
          tunnel: [w197] -> w180 mode=indexing
          shift-right: [w198] -> w179
          shift-left: w178 -> [w199]
          tunnel: w182 -> [w194] mode=indexing
          tunnel: w181 -> [w193]
          n72 = call <vilib>:"Get Type Information.vi"("error in (no error)"=w193, "variant"=w194) -> ("name"=w190:string)  [unwired: 5 in, 4 out]
          n73 = call "Set StateName.vi"("StateName"=w190, "SMO"=w189) -> ("error out"=w191:errorcluster, "SMO out"=w192:refnum<class "Instrument.lvclass">)  [unwired: 8 in]
          n74 = Scan From String(input string=w190, default 1=Instrument_Types--enum."DAQ" ("Type")) -> (output 1=w195:T8)  [unwired: 3 in, 3 out]
          n75 = call "Cast Instrument to Instrument Type.vi"("error in (no error)"=w191, "Type"=w195, "Instrument in"=w192, "Instrument Classes"=w199) -> ("error out"=w197:errorcluster, "Instrument Classes out"=w198:T13)  [unwired: 5 in, 1 out]
        }
        n76 = Bundle By Name(cluster=w185, "Instruments"=w179) -> (w186:T14)
        n77 = Merge Errors(w177, w180) -> (w184:errorcluster)
        n78 = call <vilib>:"Add State(s) to Queue__jki_lib_state_machine.vi"("State(s) in (\"\")"=w188) -> ("States Out"=w187:string)  [unwired: 14 in]
      }
      frame "Data: Disable Unsupported Instruments" {
        # "Do not put any code in this frame.\n(It is a separator no-op. You can make a copy of this frame to create a new Data frame)"
        n79 = Unbundle By Name(w209) -> ("Instruments"=w201:T13)
        n80 = call <vilib>:"Get Cluster Information.vi"("variant"=w201) -> ("error out"=w206:errorcluster, "cluster elements"=w207:variant[])  [unwired: 9 in]
        n81 = Cluster To Array(cluster=w201) -> (array=w208:refnum<class "Instrument.lvclass">[])
        n82 = for {
          tunnel: w208 -> [w219] mode=indexing
          tunnel: [w224] -> w205 mode=indexing
          shift-right: [w225] -> w200
          shift-left: w201 -> [w226]
          tunnel: w207 -> [w221] mode=indexing
          tunnel: w206 -> [w220]
          tunnel: string[] ["Lockin", "Amplifier", "Level", "VNA", "Source"] ("element") -> [w216]
          n83 = call <vilib>:"Get Type Information.vi"("error in (no error)"=w220, "variant"=w221) -> ("name"=w215:string)  [unwired: 5 in, 4 out]
          n84 = Search 1D Array(1D array=w216, element=w215) -> (index of element=w213:i32)  [unwired: 1 in]
          n85 = Greater Or Equal To 0?(x=w213) -> (x >= 0?=w214:bool)
          n86 = case shown="True" w214 {
            tunnel: w219 -> [w227 w231]
            tunnel: [w227 w230] -> w218
            tunnel: [_ w229] -> w217
            frame False {
            }
            frame True {
              n87 = call "Set IsConfigured.vi"("IsConfigured?"=FALSE, "SMO"=w231) -> ("error out"=w229:errorcluster, "SMO out"=w230:refnum<class "Instrument.lvclass">)  [unwired: 8 in]
            }
          }
          n88 = Scan From String(input string=w215, default 1=Instrument_Types--enum."DAQ" ("Type")) -> (output 1=w222:T8)  [unwired: 3 in, 3 out]
          n89 = call "Cast Instrument to Instrument Type.vi"("error in (no error)"=w217, "Type"=w222, "Instrument in"=w218, "Instrument Classes"=w226) -> ("error out"=w224:errorcluster, "Instrument Classes out"=w225:T13)  [unwired: 5 in, 1 out]
        }
        n90 = Bundle By Name(cluster=w209, "Instruments"=w200) -> (w210:T14)
        n91 = Merge Errors(w203, w205) -> (w202:errorcluster)
        n92 = call <vilib>:"Add State(s) to Queue__jki_lib_state_machine.vi"("State(s) in (\"\")"=w212) -> ("States Out"=w211:string)  [unwired: 14 in]
      }
      frame "Data: Open Instruments" {
        # "Do not put any code in this frame.\n(It is a separator no-op. You can make a copy of this frame to create a new Data frame)"
        n93 = Unbundle By Name(w240) -> ("Instruments"=w234:T13)
        n94 = call <vilib>:"Get Cluster Information.vi"("variant"=w234) -> ("error out"=w235:errorcluster, "cluster elements"=w236:variant[])  [unwired: 9 in]
        n95 = Cluster To Array(cluster=w234) -> (array=w237:refnum<class "Instrument.lvclass">[])
        n96 = for {
          tunnel: w237 -> [w247] mode=indexing
          tunnel: [w253] -> w232 mode=indexing
          shift-right: [w256] -> w233
          shift-left: w234 -> [w257]
          tunnel: w236 -> [w250] mode=indexing
          tunnel: w235 -> [w248]
          n97 = call <vilib>:"Get Type Information.vi"("error in (no error)"=w248, "variant"=w250) -> ("name"=w249:string)  [unwired: 5 in, 4 out]
          n98 = call "Get IsConfigured.vi"("SMO"=w247) -> ("error out"=w244:errorcluster, "IsConfigured?"=w245:bool, "SMO out"=w246:refnum<class "Instrument.lvclass">)  [unwired: 8 in]
          n99 = case shown="True" w245 {
            tunnel: [_ w262] -> w254
            tunnel: w246 -> [w258 w261]
            tunnel: [w258 w260] -> w255
            tunnel: w244 -> [_ w259]
            frame False {
            }
            frame True {
              n100 = call-dynamic "Open.vi"("error in (no error)"=w259, "Instrument in"=w261) -> ("error out"=w262:errorcluster, "Instrument out"=w260:refnum<class "Instrument.lvclass">)  [unwired: 8 in]
            }
          }
          n101 = Scan From String(input string=w249, default 1=Instrument_Types--enum."DAQ" ("Type")) -> (output 1=w251:T8)  [unwired: 3 in, 3 out]
          n102 = call "Cast Instrument to Instrument Type.vi"("error in (no error)"=w254, "Type"=w251, "Instrument in"=w255, "Instrument Classes"=w257) -> ("error out"=w253:errorcluster, "Instrument Classes out"=w256:T13)  [unwired: 5 in, 1 out]
        }
        n103 = Bundle By Name(cluster=w240, "Instruments"=w233) -> (w241:T14)
        n104 = Merge Errors(w238, w232) -> (w239:errorcluster)
        n105 = call <vilib>:"Add State(s) to Queue__jki_lib_state_machine.vi"("State(s) in (\"\")"=w243) -> ("States Out"=w242:string)  [unwired: 14 in]
      }
      frame "Data: Configure Magnet Type" {
        # "Do not put any code in this frame.\n(It is a separator no-op. You can make a copy of this frame to create a new Data frame)"
        n106 = Unbundle By Name(w263) -> ("Instruments.Magnet"=w268:refnum<class "Instrument.Cryostat.lvclass">)
        n107 = call <vilib>:"Get LV Class Name.vi"("error in (no error)"=w272, "object"=w268) -> ("error out"=w266:errorcluster, "class name"=w276:string)  [unwired: 8 in]
        n108 = Match Pattern(string=w276, regular expression="VRM") -> (offset past match=w274:i32)  [unwired: 1 in, 3 out]
        n109 = Greater Or Equal To 0?(x=w274) -> (x >= 0?=w264:bool)
        n110 = Select(t="Vector Magnet" ("new element/subarray"), s=w264, f="Magnet" ("element")) -> (s? t:f=w269:string)
        n111 = call "Set StateName.vi"("error in (no error)"=w266, "StateName"=w269, "SMO"=w268) -> ("error out"=w265:errorcluster, "SMO out"=w267:refnum<class "Instrument.Cryostat.lvclass">)  [unwired: 7 in]
        n112 = Bundle By Name(cluster=w263, "Instruments.Magnet"=w267) -> (w273:T14)
        n113 = call <vilib>:"Add State(s) to Queue__jki_lib_state_machine.vi"("State(s) in (\"\")"=w278) -> ("States Out"=w277:string)  [unwired: 14 in]
      }
      frame "Data: Close Instruments" {
        # "Data: Close Instruments\n(Close Instruments that are explicitly opened by this VI)"
        n114 = Unbundle By Name(w284) -> ("Instruments"=w281:T13)
        n115 = call <vilib>:"Get Cluster Information.vi"("variant"=w281) -> ("error out"=w279:errorcluster, "cluster elements"=w280:variant[])  [unwired: 9 in]
        n116 = Cluster To Array(cluster=w281) -> (array=w287:refnum<class "Instrument.lvclass">[])
        n117 = for {
          tunnel: w287 -> [w294] mode=indexing
          tunnel: [w300] -> w288 mode=indexing
          shift-right: [w303] -> w286
          shift-left: w281 -> [w304]
          tunnel: w280 -> [w297] mode=indexing
          tunnel: w279 -> [w295]
          n118 = call <vilib>:"Get Type Information.vi"("error in (no error)"=w295, "variant"=w297) -> ("name"=w296:string)  [unwired: 5 in, 4 out]
          n119 = call "Get IsConfigured.vi"("SMO"=w294) -> ("error out"=w291:errorcluster, "IsConfigured?"=w293:bool, "SMO out"=w292:refnum<class "Instrument.lvclass">)  [unwired: 8 in]
          n120 = case shown="True" w293 {
            tunnel: [w305 w309] -> w301
            tunnel: w292 -> [w306 w308]
            tunnel: [w306 w307] -> w302
            tunnel: w291 -> [w305 _]
            frame False {
            }
            frame True {
              n121 = call-dynamic "Close.vi"("Instrument in"=w308) -> ("error out"=w309:errorcluster, "Instrument out"=w307:refnum<class "Instrument.lvclass">)  [unwired: 9 in]
            }
          }
          n122 = Scan From String(input string=w296, default 1=Instrument_Types--enum."DAQ" ("Type")) -> (output 1=w298:T8)  [unwired: 3 in, 3 out]
          n123 = call "Cast Instrument to Instrument Type.vi"("error in (no error)"=w301, "Type"=w298, "Instrument in"=w302, "Instrument Classes"=w304) -> ("error out"=w300:errorcluster, "Instrument Classes out"=w303:T13)  [unwired: 5 in, 1 out]
        }
        n124 = Bundle By Name(cluster=w284, "Instruments"=w286) -> (w283:T14)
        n125 = Merge Errors(w285, w288) -> (w282:errorcluster)
        n126 = call <vilib>:"Add State(s) to Queue__jki_lib_state_machine.vi"("State(s) in (\"\")"=w290) -> ("States Out"=w289:string)  [unwired: 14 in]
      }
      frame "Data: UI Stop" {
        # "Data: UI Stop\n(Used to record when stop signal comes from UI (front panel stop or panel close)"
        n127 = Scan From String(input string=w312, default 1=FALSE) -> (output 1=w311:bool)  [unwired: 3 in, 3 out]
        n128 = Bundle By Name(cluster=w313, "UI stop"=w311) -> (w314:T14)
        n129 = call <vilib>:"Add State(s) to Queue__jki_lib_state_machine.vi"("State(s) in (\"\")"=w317) -> ("States Out"=w316:string)  [unwired: 14 in]
      }
      frame "Data: Cleanup" {
        # "Cleanup any data and references, here.\n(this is called automatically, by the Macro: Exit)"
        n130 = Unbundle By Name(w332) -> ("Transport"=w336:refnum<class "Transport.lvclass">, "Execution:State"=w329:T7, "C.E."=w328:refnum<class "Control Experiment.lvclass">, "Instruments"=w327:T13, "Core.Current VI Reference"=w334:refnum<vi>)
        n131 = case shown="\"Run top level\"" w329 {
          tunnel: [w341 w346] -> w326
          tunnel: w328 -> [w341 w345]
          tunnel: w324 -> [w339 w343]
          tunnel: [w339 w344] -> w323
          tunnel: w327 -> [w340 w342]
          tunnel: [w340 w342] -> w325
          frame Default {
          }
          frame "Run top level" {
            n132 = call "Close Dictionary.vi"("error in (no error)"=w343, "Control Experiment in"=w345) -> ("error out"=w344:errorcluster, "Control Experiment out"=w346:refnum<class "Control Experiment.lvclass">)  [unwired: 8 in]
          }
        }
        n133 = call "Write Instruments.vi"("error in (no error)"=w323, "Instruments"=w325, "Control Experiment in"=w326) -> ("error out"=w330:errorcluster, "Control Experiment out"=w331:refnum<class "Control Experiment.lvclass">)  [unwired: 7 in]
        n134 = call "Write Dependencies.vi"("error in (no error)"=w330, "Control Experiment"=w331, "Transport in"=w336) -> ("error out"=w319:errorcluster, "Transport out"=w321:refnum<class "Transport.lvclass">)  [unwired: 7 in]
        n135 = call "Send RunningStatus Notifier.vi"("error in (no error)"=w319, "Running?"=FALSE, "Transport in"=w321) -> ("error out"=w318:errorcluster, "Transport out"=w320:refnum<class "Transport.lvclass">)  [unwired: 7 in]
        n136 = Bundle By Name(cluster=w332, "Transport"=w320) -> (w335:T14)
        n137 = Close Reference(reference=w334, error in (no error)=w318) -> (error out=w333:errorcluster)
        n138 = call <vilib>:"Add State(s) to Queue__jki_lib_state_machine.vi"("State(s) in (\"\")"=w338) -> ("States Out"=w337:string)  [unwired: 14 in]
      }
      frame "---------- UI ----------" {
        # "Do not put any code in this frame.\n(It is a separator no-op. You can make a copy of this frame to create a new UI frame)"
        n139 = call <vilib>:"Add State(s) to Queue__jki_lib_state_machine.vi"("State(s) in (\"\")"=w350) -> ("States Out"=w349:string)  [unwired: 14 in]
      }
      frame "UI: Initialize" {
        # "Initialize the User Interface, here.\n(this is called automatically, by the Macro: Init)"
        n140 = call <userlib>:"Tick Count (ms)__ogtk.vi"("error in (no error)"=w359) -> ("error out"=w358:errorcluster, "millisecond timer value"=w357:u32)  [unwired: 9 in]
        n141 = Unbundle By Name(w352) -> ("Run Time System?"=w351:bool)
        n142 = call <userlib>:"Fit VI window to Largest Dec__ogtk.vi"("error in (no error)"=w358, "border spacing (2 px)"=0) -> ("error out"=w354:errorcluster)  [unwired: 4 in, 1 out]
        n143 = local read "Emergency Stop Visible?"() -> (w353:bool)
        n144 = invoke on="stop" class="Bool (strict)" method="Reinit To Default"() -> ()  [unwired: 3 in, 3 out]
        n145 = property on="Emergency Stop Visible?" class="Bool (strict)"("Val(Sgnl)"=w353) -> ()  [unwired: 2 in, 2 out]
        n146 = property on="Start" class="Bool (strict)"("Visible"=w351) -> ()  [unwired: 2 in, 2 out]
        n147 = Bundle By Name(cluster=w352, "ms [0]"=w357, "ms [i]"=w357) -> (w355:T14)
        n148 = call <vilib>:"Add State(s) to Queue__jki_lib_state_machine.vi"("State(s) in (\"\")"=w361) -> ("States Out"=w360:string)  [unwired: 14 in]
      }
      frame "UI: Cursor Set" {
        # "Argument"
        # "Set and Unset Cursor Busy.\n(Usage: \"UI: Cursor Set >> Busy|Idle\")"
        n149 = case shown="\"Idle\", Default" w362 {
          tunnel: w364 -> [w369 w371]
          tunnel: [w368 w370] -> w363
          frame "Idle", Default {
            n150 = call <vilib>:"Unset Busy.vi"("error in (no error)"=w369) -> ("error out"=w368:errorcluster)  [unwired: 10 in]
          }
          frame "Busy" {
            n151 = call <vilib>:"Set Busy.vi"("error in (no error)"=w371) -> ("error out"=w370:errorcluster)  [unwired: 9 in, 1 out]
          }
        }
        n152 = call <vilib>:"Add State(s) to Queue__jki_lib_state_machine.vi"("State(s) in (\"\")"=w367) -> ("States Out"=w366:string)  [unwired: 14 in]
      }
      frame "UI: Emergency Stop Visible" {
        # "Do not put any code in this frame.\n(It is a separator no-op. You can make a copy of this frame to create a new UI frame)"
        n153 = Scan From String(input string=w374, default 1=FALSE) -> (output 1=w372:bool)  [unwired: 3 in, 3 out]
        n154 = property on="Emergency Stop 1" class="Bool"("Visible"=w372) -> ()  [unwired: 2 in, 2 out]
        n155 = property on="Emergency Stop 2" class="Bool"("Visible"=w372) -> ()  [unwired: 2 in, 2 out]
        n156 = property on="Emergency Stop 3" class="Bool"("Visible"=w372) -> ()  [unwired: 2 in, 2 out]
        n157 = property on="Emergency Stop 4" class="Bool"("Visible"=w372) -> ()  [unwired: 2 in, 2 out]
        n158 = call <vilib>:"Add State(s) to Queue__jki_lib_state_machine.vi"("State(s) in (\"\")"=w378) -> ("States Out"=w377:string)  [unwired: 14 in]
      }
      frame "UI: Update Timer" {
        n159 = Unbundle By Name(w390) -> ("ms [0]"=w391:u32)
        n160 = call <userlib>:"Tick Count (ms)__ogtk.vi"("error in (no error)"=w381) -> ("error out"=w380:errorcluster, "millisecond timer value"=w385:u32)  [unwired: 9 in]
        n161 = Subtract(x=w385, y=w391) -> (x-y=w388:u32)
        n162 = call <userlib>:"MGI Milliseconds Since Last Call.vi"("Error In"=w380) -> ("ms"=→"time b/w points (ms)":u32, "Error Out"=w386:errorcluster)  [unwired: 5 in]
        n163 = To Double Precision Float(number=w388) -> (double precision float=w384:dbl)
        n164 = To Double Precision Float(number=u32 1000 ("x")) -> (double precision float=w383:dbl)
        n165 = Bundle By Name(cluster=w390, "ms [i]"=w385) -> (w389:T14)
        n166 = Divide(x=w384, y=w383) -> (x/y=w392:dbl)
        n167 = To Long Integer(number=w392) -> (32bit integer=→"elapsed time (s)":i32)
        n168 = call <vilib>:"Add State(s) to Queue__jki_lib_state_machine.vi"("State(s) in (\"\")"=w394) -> ("States Out"=w393:string)  [unwired: 14 in]
      }
      frame "UI: Update Status" {
        # "Do not put any code in this frame.\n(It is a separator no-op. You can make a copy of this frame to create a new UI frame)"
        n169 = local read "Instrument Status"() -> (w397:string)
        n170 = To Lower Case(string=w396) -> (all lower case string=w404:string)
        n171 = Empty String/Path?(string/path=w397) -> (empty?=w395:bool)
        n172 = Equal?(x=w404, y="reset") -> (x = y?=w403:bool)
        n173 = Format Into String(format string="%s, %s", w397, w396) -> (resulting string=w399:string)  [unwired: 2 in, 1 out]
        n174 = Select(t=w396, s=w395, f=w399) -> (s? t:f=w398:string)
        n175 = Select(t="", s=w403, f=w398) -> (s? t:f=→"Instrument Status":string)
        n176 = call <vilib>:"Add State(s) to Queue__jki_lib_state_machine.vi"("State(s) in (\"\")"=w409) -> ("States Out"=w408:string)  [unwired: 14 in]
      }
      frame "UI: Update Graph Axis Labels" {
        w412 = "sweep (V)" ("string")
        n177 = control-ref of="AO"() -> (w414:refnum<vi>)
        n178 = control-ref of="AI"() -> (w413:refnum<vi>)
        n179 = control-ref of="2 Terminal"() -> (w418:refnum<vi>)
        n180 = control-ref of="4 Terminal"() -> (w417:refnum<vi>)
        n181 = control-ref of="Lockin (X)"() -> (w427:refnum<vi>)
        n182 = control-ref of="Lockin (Y)"() -> (w426:refnum<vi>)
        n183 = control-ref of="Resistance"() -> (w424:refnum<vi>)
        n184 = control-ref of="Conductance"() -> (w419:refnum<vi>)
        n185 = local read "Units"() -> (w422:enum16{"ohms & siemens", "h/e2 & e2/h"})
        n186 = case shown="\"h/e2 & e2/h\"" w422 {
          tunnel: ["R (ohms)" "R (h/e2)"] -> w421
          tunnel: ["G (siemens)" "G (e2/h)"] -> w420
          frame "ohms & siemens", Default {
          }
          frame "h/e2 & e2/h" {
          }
        }
        n187 = property on="Property Node" class="XYGraph (strict)"(reference=w418, "XScale.NameLbl.Text"=w412) -> (error out=w415:errorcluster)  [unwired: 1 in, 1 out]
        n188 = property on="Property Node" class="XYGraph (strict)"(reference=w417, "XScale.NameLbl.Text"=w412) -> (error out=w416:errorcluster)  [unwired: 1 in, 1 out]
        n189 = property on="Property Node" class="XYGraph (strict)"(reference=w427, "XScale.NameLbl.Text"=w412) -> (error out=w431:errorcluster)  [unwired: 1 in, 1 out]
        n190 = property on="Property Node" class="XYGraph (strict)"(reference=w426, "XScale.NameLbl.Text"=w412) -> (error out=w432:errorcluster)  [unwired: 1 in, 1 out]
        n191 = property on="Property Node" class="XYGraph (strict)"(reference=w424, "XScale.NameLbl.Text"=w412, "YScale.NameLbl.Text"=w421) -> (error out=w433:errorcluster)  [unwired: 1 in, 1 out]
        n192 = property on="Property Node" class="XYGraph (strict)"(reference=w419, "XScale.NameLbl.Text"=w412, "YScale.NameLbl.Text"=w420) -> (error out=w423:errorcluster)  [unwired: 1 in, 1 out]
        n193 = property on="Property Node" class="XYGraph (strict)"(reference=w414, "XScale.NameLbl.Text"=w412) -> (error out=w410:errorcluster)  [unwired: 1 in, 1 out]
        n194 = property on="Property Node" class="XYGraph (strict)"(reference=w413, "XScale.NameLbl.Text"=w412) -> (error out=w411:errorcluster)  [unwired: 1 in, 1 out]
        n195 = Merge Errors(w410, w411, w415, w416, w431, w432, w433, w423, w429) -> (w428:errorcluster)
        n196 = call <vilib>:"Clear Errors.vi"("error in (no error)"=w428) -> ("error out"=w430:errorcluster)  [unwired: 5 in, 1 out]
        n197 = call <vilib>:"Add State(s) to Queue__jki_lib_state_machine.vi"("State(s) in (\"\")"=w435) -> ("States Out"=w434:string)  [unwired: 14 in]
      }
      frame "UI: Update Lockin Graph Legend" {
        n198 = Unbundle By Name(w448) -> ("Results (Dictionary)"=w445:cluster{"key":string, "value":dbl}[])
        n199 = call <userlib>:"Parse Results (all).vi"("Type"=Results_Type--Enum."X", "error in (no error)"=w446, "Results (Dictionary)"=w445) -> ("error out"=w447:errorcluster, "Label"=w442:string[])  [unwired: 5 in, 2 out]
        n200 = Array Size(array=w442) -> (size(s)=w443:i32)
        n201 = for {
          tunnel: w447 -> [w460]
          tunnel: w442 -> [w456] mode=indexing
          tunnel: w443 -> [w455]
          tunnel: [w454] -> w441 mode=indexing
          tunnel: [w453] -> w440 mode=indexing
          i -> [w459]
          n202 = control-ref of="Lockin (X)"() -> (w457:refnum<vi>)
          n203 = property on="Property Node" class="XYGraph (strict)"(reference=w457, error in=w460, "Active Plot"=w459, "Plot.Plot Name"=w456, "LegPlotMin"=w455) -> (error out=w453:errorcluster)  [unwired: 1 out]
          n204 = control-ref of="Lockin (Y)"() -> (w458:refnum<vi>)
          n205 = property on="Property Node" class="XYGraph (strict)"(reference=w458, "Active Plot"=w459, "Plot.Plot Name"=w456, "LegPlotMin"=w455) -> (error out=w454:errorcluster)  [unwired: 1 in, 1 out]
        }
        n206 = Merge Errors(w441, w440) -> (w444:errorcluster)
        n207 = call <vilib>:"Clear Errors.vi"("error in (no error)"=w444) -> ("error out"=w450:errorcluster)  [unwired: 5 in, 1 out]
        n208 = call <vilib>:"Add State(s) to Queue__jki_lib_state_machine.vi"("State(s) in (\"\")"=w452) -> ("States Out"=w451:string)  [unwired: 14 in]
      }
      frame "UI: Update Wfm Graph Legend" {
        n209 = Unbundle By Name(w469) -> ("AO Waveforrm"=w466:waveform(dbl)[], "AI Waveform"=w465:waveform(dbl)[])
        n210 = Array Size(array=w465) -> (size(s)=w464:i32)
        n211 = Array Size(array=w466) -> (size(s)=w467:i32)
        n212 = for {
          N: w467 -> [w480]
          tunnel: [w485] -> w462 mode=indexing
          i -> [w484]
          n213 = Increment(x=w484) -> (x+1=w481:i32)
          n214 = control-ref of="AO"() -> (w486:refnum<vi>)
          n215 = Format Into String(format string="AO %d", w481) -> (resulting string=w482:string)  [unwired: 2 in, 1 out]
          n216 = property on="Property Node" class="XYGraph (strict)"(reference=w486, "Active Plot"=w484, "Plot.Plot Name"=w482, "LegPlotMin"=w480) -> (error out=w485:errorcluster)  [unwired: 1 in, 1 out]
        }
        n217 = for {
          N: w464 -> [w474]
          tunnel: [w479] -> w463 mode=indexing
          i -> [w478]
          n218 = Increment(x=w478) -> (x+1=w475:i32)
          n219 = control-ref of="AI"() -> (w473:refnum<vi>)
          n220 = Format Into String(format string="AI %d", w475) -> (resulting string=w476:string)  [unwired: 2 in, 1 out]
          n221 = property on="Property Node" class="XYGraph (strict)"(reference=w473, "Active Plot"=w478, "Plot.Plot Name"=w476, "LegPlotMin"=w474) -> (error out=w479:errorcluster)  [unwired: 1 in, 1 out]
        }
        n222 = Merge Errors(w462, w463, w461) -> (w468:errorcluster)
        n223 = call <vilib>:"Clear Errors.vi"("error in (no error)"=w468) -> ("error out"=w470:errorcluster)  [unwired: 5 in, 1 out]
        n224 = call <vilib>:"Add State(s) to Queue__jki_lib_state_machine.vi"("State(s) in (\"\")"=w472) -> ("States Out"=w471:string)  [unwired: 14 in]
      }
      frame "UI: Update R G Graph Legend" {
        n225 = local read "Resistance"() -> (w502:cluster{"X-array":dbl[], "Y-array":dbl[]}[])
        n226 = local read "Conductance"() -> (w503:cluster{"X-array":dbl[], "Y-array":dbl[]}[])
        n227 = Array Size(array=w502) -> (size(s)=w491:i32)
        n228 = Array Size(array=w503) -> (size(s)=w501:i32)
        n229 = Quotient & Remainder(x=w491, y=2) -> (floor(x/y)=w488:i32)  [unwired: 1 out]
        n230 = Quotient & Remainder(x=w501, y=2) -> (floor(x/y)=w495:i32)  [unwired: 1 out]
        n231 = Greater?(x=w488, y=1) -> (0:w487:bool)
        n232 = Greater?(x=w495, y=1) -> (0:w498:bool)
        n233 = case shown="True" w487 {
          tunnel: string[] ["R2T", "R4T"] -> [w511 w514]
          tunnel: [w511 w512] -> w490
          tunnel: w488 -> [_ w513]
          frame False {
          }
          frame True {
            n234 = for {
              N: w513 -> [_]
              tunnel: w514 -> [w517]
              tunnel: [w515] -> w512 mode=concatenating
              i -> [w519]
              n235 = call <vilib>:"Space Constant.vi"() -> ("String"=w518:string)
              n236 = Format Into String(initial string=w518, w519) -> (resulting string=w516:string)  [unwired: 2 in, 1 out]
              n237 = for {
                tunnel: w517 -> [w522] mode=indexing
                tunnel: w516 -> [w521]
                tunnel: [w520] -> w515 mode=indexing
                n238 = Concatenate Strings(w522, w521) -> (w520:string)
              }
            }
          }
        }
        n239 = case shown="False" w498 {
          tunnel: string[] ["G2T", "G4T"] -> [w523 w526]
          tunnel: [w523 w524] -> w499
          tunnel: w495 -> [_ w525]
          frame False {
          }
          frame True {
            n240 = for {
              N: w525 -> [_]
              tunnel: w526 -> [w529]
              tunnel: [w527] -> w524 mode=concatenating
              i -> [w531]
              n241 = call <vilib>:"Space Constant.vi"() -> ("String"=w530:string)
              n242 = Format Into String(initial string=w530, w531) -> (resulting string=w528:string)  [unwired: 2 in, 1 out]
              n243 = for {
                tunnel: w529 -> [w534] mode=indexing
                tunnel: w528 -> [w533]
                tunnel: [w532] -> w527 mode=indexing
                n244 = Concatenate Strings(w534, w533) -> (w532:string)
              }
            }
          }
        }
        n245 = for {
          N: w501 -> [w542]
          tunnel: [w543] -> w504 mode=indexing
          tunnel: w499 -> [w540] mode=indexing
          i -> [w541]
          n246 = control-ref of="Conductance"() -> (w544:refnum<vi>)
          n247 = property on="Property Node" class="XYGraph (strict)"(reference=w544, "Active Plot"=w541, "Plot.Plot Name"=w540, "LegPlotMin"=w542) -> (error out=w543:errorcluster)  [unwired: 1 in, 1 out]
        }
        n248 = for {
          N: w491 -> [w537]
          tunnel: [w539] -> w505 mode=indexing
          tunnel: w490 -> [w535] mode=indexing
          i -> [w538]
          n249 = control-ref of="Resistance"() -> (w536:refnum<vi>)
          n250 = property on="Property Node" class="XYGraph (strict)"(reference=w536, "Active Plot"=w538, "Plot.Plot Name"=w535, "LegPlotMin"=w537) -> (error out=w539:errorcluster)  [unwired: 1 in, 1 out]
        }
        n251 = Merge Errors(w504, w505, w494) -> (w506:errorcluster)
        n252 = call <vilib>:"Add State(s) to Queue__jki_lib_state_machine.vi"("State(s) in (\"\")"=w510) -> ("States Out"=w509:string)  [unwired: 14 in]
        n253 = call <vilib>:"Clear Errors.vi"("error in (no error)"=w506) -> ("error out"=w508:errorcluster)  [unwired: 5 in, 1 out]
      }
      frame "UI: Update AO AI Graphs" {
        n254 = Unbundle By Name(w557) -> ("Sweep Value"=w545:dbl, "AO Waveforrm"=w551:waveform(dbl)[], "AI Waveform"=w552:waveform(dbl)[])  [unwired: 1 out]
        n255 = To Lower Case(string=w553) -> (all lower case string=w554:string)
        n256 = Equal?(x=w554, y="reset") -> (x = y?=w548:bool)
        n257 = for {
          tunnel: w551 -> [w561] mode=indexing
          tunnel: [w560] -> w547 mode=indexing
          n258 = Unbundle By Name(w561) -> ("Y"=w562:dbl[])
          n259 = Index Array(array=w562) -> (element=w560:dbl)  [unwired: 1 in]
        }
        n260 = for {
          tunnel: w552 -> [w564] mode=indexing
          tunnel: [w563] -> w546 mode=indexing
          n261 = Unbundle By Name(w564) -> ("Y"=w565:dbl[])
          n262 = Index Array(array=w565) -> (element=w563:dbl)  [unwired: 1 in]
        }
        n263 = call "Graph Lockin vs Parameter.vi"("reset?"=w548, "Y"=w547, "X"=w545) -> ("Data vs Parameter"=→"AO":cluster{dbl[], dbl[]}[])  [unwired: 8 in]
        n264 = call "Graph Lockin vs Parameter.vi"("reset?"=w548, "Y"=w546, "X"=w545) -> ("Data vs Parameter"=→"AI":cluster{dbl[], dbl[]}[])  [unwired: 8 in]
        n265 = call <vilib>:"Add State(s) to Queue__jki_lib_state_machine.vi"("State(s) in (\"\")"=w559) -> ("States Out"=w558:string)  [unwired: 14 in]
      }
      frame "UI: Update Lockin Graphs" {
        # "results"
        n266 = Unbundle By Name(w576) -> ("Sweep Value"=w566:dbl, "Results (Dictionary)"=w582:cluster{"key":string, "value":dbl}[])  [unwired: 1 out]
        n267 = To Lower Case(string=w573) -> (all lower case string=w574:string)
        n268 = Equal?(x=w574, y="reset") -> (x = y?=w567:bool)
        n269 = call <userlib>:"Parse Results (all).vi"("Type"=Results_Type--Enum."X", "error in (no error)"=w571, "Results (Dictionary)"=w582) -> ("error out"=w578:errorcluster, "Data"=w569:dbl[], "Results (Dictionary)"=w579:cluster{"key":string, "value":dbl}[])  [unwired: 5 in, 1 out]
        n270 = call <userlib>:"Parse Results (all).vi"("Type"=Results_Type--Enum."Y", "error in (no error)"=w578, "Results (Dictionary)"=w579) -> ("error out"=w577:errorcluster, "Data"=w568:dbl[])  [unwired: 5 in, 2 out]
        n271 = call "Graph Lockin vs Parameter.vi"("reset?"=w567, "Y"=w569, "X"=w566) -> ("Data vs Parameter"=→"Lockin (X)":cluster{dbl[], dbl[]}[])  [unwired: 8 in]
        n272 = call "Graph Lockin vs Parameter.vi"("reset?"=w567, "Y"=w568, "X"=w566) -> ("Data vs Parameter"=→"Lockin (Y)":cluster{dbl[], dbl[]}[])  [unwired: 8 in]
        n273 = call <vilib>:"Add State(s) to Queue__jki_lib_state_machine.vi"("State(s) in (\"\")"=w584) -> ("States Out"=w583:string)  [unwired: 14 in]
      }
      frame "UI: Update R G Graphs" {
        # "Do not put any code in this frame.\n(It is a separator no-op. You can make a copy of this frame to create a new UI frame)"
        n274 = Unbundle By Name(w591) -> ("Amplitude"=w590:dbl[], "C.E."=w589:refnum<class "Control Experiment.lvclass">)
        n275 = call "Get Channel Indices.vi"("Control Experiment in"=w589) -> ("Indices"=w588:T16)  [unwired: 8 in, 2 out]
        n276 = local read "Lockin (Y)"() -> (w592:cluster{"Wavenumber":dbl[], "Data":dbl[]}[])
        n277 = local read "Lockin (X)"() -> (w593:cluster{"Wavenumber":dbl[], "Data":dbl[]}[])
        n278 = case shown="\"h/e2 & e2/h\"" "Units" {
          tunnel: [1.0 ("Siemens/(e2/h)") w601] -> w596
          frame "ohms & siemens", Default {
          }
          frame "h/e2 & e2/h" {
            w601 = 3.874046e-05  # Siemens/(e2/h)
          }
        }
        n279 = call "Graph R and G vs Parameter.vi"("indices"=w588, "AO Amp (V)"=w590, "Y vs Parameter"=w592, "X vs Parameter"=w593) -> ("G(Siemens) vs Parameter"=w595:cluster{"X-array":dbl[], dbl[]}[], "R(Ohms) vs Parameter"=w594:cluster{"X-array":dbl[], dbl[]}[])  [unwired: 6 in]
        n280 = call-poly <vilib>:"Multiply.vi"("y (1)"=w596, "XY-data"=w594) -> ("XY-data out"=→"Resistance":cluster{"X-array":dbl[], "Y-array":dbl[]}[])  [unwired: 8 in, 1 out]
        n281 = call-poly <vilib>:"Divide.vi"("y (1)"=w596, "XY-data"=w595) -> ("XY-data out"=→"Conductance":cluster{"X-array":dbl[], "Y-array":dbl[]}[])  [unwired: 8 in, 1 out]
        n282 = call <vilib>:"Add State(s) to Queue__jki_lib_state_machine.vi"("State(s) in (\"\")"=w599) -> ("States Out"=w598:string)  [unwired: 14 in]
      }
      frame "UI: Update Graphs from wfm" {
        # "Do not put any code in this frame.\n(It is a separator no-op. You can make a copy of this frame to create a new UI frame)"
        n283 = local read "Sweep Channels"() -> (w612:T2)
        n284 = Unbundle By Name(w614) -> ("Sweep_AO"=w609:waveform(dbl)[], "Sweep_AI"=w608:waveform(dbl)[], "Sweep_X"=w607:waveform(dbl)[], "Sweep_Y"=w606:waveform(dbl)[])  [unwired: 1 out]
        n285 = for {
          tunnel: [w630] -> w611
          tunnel: w612 -> [w633] mode=indexing
          stop <- w632 stop-if-true
          # "find the 1st enabled channel"
          n286 = Unbundle By Name(w633) -> ("Enable?"=w632:bool, "Channel"=w631:u16)
          n287 = Decrement(x=w631) -> (x-1=w630:u16)
        }
        n288 = Index Array(array=w609, index=w611) -> (element=w613:waveform(dbl))
        n289 = Unbundle By Name(w613) -> ("Y"=w605:dbl[])
        n290 = for {
          tunnel: w605 -> [w626]
          tunnel: w608 -> [w628] mode=indexing
          tunnel: [w627] -> w602 mode=indexing
          n291 = Unbundle By Name(w628) -> ("Y"=w629:dbl[])
          n292 = call <vilib>:"Initialize.vi"("Y-array"=w629, "X-array"=w626) -> ("XY-data out"=w627:cluster{"X-array":dbl[], "Y-array":dbl[]})  [unwired: 8 in, 1 out]
        }
        n293 = for {
          tunnel: w605 -> [w634]
          tunnel: w609 -> [w636] mode=indexing
          tunnel: [w635] -> w610 mode=indexing
          n294 = Unbundle By Name(w636) -> ("Y"=w637:dbl[])
          n295 = call <vilib>:"Initialize.vi"("Y-array"=w637, "X-array"=w634) -> ("XY-data out"=w635:cluster{"X-array":dbl[], "Y-array":dbl[]})  [unwired: 8 in, 1 out]
        }
        n296 = for {
          tunnel: w605 -> [w618]
          tunnel: w606 -> [w620] mode=indexing
          tunnel: [w619] -> w604 mode=indexing
          n297 = Unbundle By Name(w620) -> ("Y"=w621:dbl[])
          n298 = call <vilib>:"Initialize.vi"("Y-array"=w621, "X-array"=w618) -> ("XY-data out"=w619:cluster{"X-array":dbl[], "Y-array":dbl[]})  [unwired: 8 in, 1 out]
        }
        n299 = for {
          tunnel: w605 -> [w622]
          tunnel: w607 -> [w624] mode=indexing
          tunnel: [w623] -> w603 mode=indexing
          n300 = Unbundle By Name(w624) -> ("Y"=w625:dbl[])
          n301 = call <vilib>:"Initialize.vi"("Y-array"=w625, "X-array"=w622) -> ("XY-data out"=w623:cluster{"X-array":dbl[], "Y-array":dbl[]})  [unwired: 8 in, 1 out]
        }
        n302 = local write "AO"(w610) -> ()
        n303 = local write "AI"(w602) -> ()
        n304 = local write "Lockin (X)"(w603) -> ()
        n305 = local write "Lockin (Y)"(w604) -> ()
        n306 = call <vilib>:"Add State(s) to Queue__jki_lib_state_machine.vi"("State(s) in (\"\")"=w617) -> ("States Out"=w616:string)  [unwired: 14 in]
      }
      frame "UI: Update IV Graphs" {
        # "Do not put any code in this frame.\n(It is a separator no-op. You can make a copy of this frame to create a new UI frame)"
        n307 = Unbundle By Name(w654) -> ("Sweep_AI"=w651:waveform(dbl)[], "Sweep_AO"=w650:waveform(dbl)[], "C.E."=w656:refnum<class "Control Experiment.lvclass">)
        n308 = call "Get Channel Indices.vi"("error in (no error)"=w646, "Control Experiment in"=w656) -> ("error out"=w645:errorcluster, "Indices"=w643:T16)  [unwired: 7 in, 1 out]
        n309 = Decrement(x=w643) -> (x-1=w642:T16)
        n310 = Unbundle By Name(w642) -> ("I-"=w657:i32, "V1+"=w655:i32, "V1-"=w641:i32, "I+"=w660:i32)
        n311 = Equal?(x=w655, y=w641) -> (x = y?=w639:bool)
        n312 = Index Array(array=w651, index #1=w657, index #2=w655, index #3=w641) -> (element #1=w644:waveform(dbl), element #2=w659:waveform(dbl), element #3=w640:waveform(dbl))
        n313 = Index Array(array=w650, index=w660) -> (element=w661:waveform(dbl))
        n314 = case shown="False" w639 {
          tunnel: w659 -> [w665 w669]
          tunnel: w640 -> [_ w668]
          tunnel: [w665 w667] -> w638
          tunnel: [_ w666] -> _
          frame True {
          }
          frame False {
            n315 = Subtract(1:w668, 2:w669) -> (0:w667:waveform(dbl), 3:w666:errorcluster)  [unwired: 1 in]
          }
        }
        n316 = Unbundle By Name(w644) -> ("Y"=w649:dbl[])
        n317 = Unbundle By Name(w638) -> ("Y"=w648:dbl[])
        n318 = Unbundle By Name(w661) -> ("Y"=w647:dbl[])
        n319 = Bundle("Y"=w648, "Y"=w649) -> (w658:cluster{"Y":dbl[], "Y":dbl[]})  [unwired: 1 in]
        n320 = Bundle("Y"=w647, "Y"=w649) -> (w662:cluster{"Y":dbl[], "Y":dbl[]})  [unwired: 1 in]
        n321 = Build Array(w658) -> (→"4 Terminal":cluster{"Y":dbl[], "Y":dbl[]}[])
        n322 = Build Array(w662) -> (→"2 Terminal":cluster{"Y":dbl[], "Y":dbl[]}[])
        n323 = call <vilib>:"Add State(s) to Queue__jki_lib_state_machine.vi"("State(s) in (\"\")"=w664) -> ("States Out"=w663:string)  [unwired: 14 in]
      }
      frame "UI: Front Panel State" {
        # "Argument"
        # "Set Front Panel Open or Closed\n(Usage: \"UI: Front Panel State >> Open|Close\")"
        n324 = Unbundle By Name(w672) -> ("Core.Current VI Reference"=w671:refnum<vi>)
        n325 = case shown="\"Maximize\", \"Maximized\"" w670 {
          tunnel: w674 -> [w682 w697 w708 w721 w734]
          tunnel: [w684 w698 w710 w723 w736] -> w673
          tunnel: w671 -> [w683 w695 w709 w722 w735]
          frame "Open", "Standard", Default {
            w677 = T5."Standard" ("State")
            n326 = property class="VI"(reference=w683, error in=w682) -> (reference out=w680:refnum<vi>, error out=w681:errorcluster, "FP.State"=w679:T5)
            n327 = Not Equal?(x=w679, y=w677) -> (x != y?=w678:bool)
            n328 = case shown="False" w678 {
              tunnel: [w688 w690] -> w684
              tunnel: w681 -> [w687 w690]
              tunnel: w680 -> [w686 _]
              tunnel: w677 -> [w685 _]
              frame True {
                n329 = invoke class="VI" method="FP.Open"(reference=w686, error in=w687, "Activate"=TRUE, "State"=w685) -> (error out=w688:errorcluster)  [unwired: 1 in, 4 out]
              }
              frame False {
              }
            }
          }
          frame "Close", "Closed" {
            n330 = property class="VI"(reference=w695, error in=w697) -> (reference out=w694:refnum<vi>, error out=w696:errorcluster, "FP.State"=w692:T5)
            n331 = Not Equal?(x=w692, y=T5."Closed" ("Front Panel Window:State")) -> (x != y?=w691:bool)
            n332 = case shown="True" w691 {
              tunnel: [w699 w702] -> w698
              tunnel: w696 -> [w699 w701]
              tunnel: w694 -> [_ w700]
              frame False {
              }
              frame True {
                n333 = invoke class="VI" method="FP.Close"(reference=w700, error in=w701) -> (error out=w702:errorcluster)  [unwired: 1 in, 2 out]
              }
            }
          }
          frame "Hidden", "Hide" {
            w703 = T5."Hidden" ("State")
            n334 = property class="VI"(reference=w709, error in=w708) -> (reference out=w706:refnum<vi>, error out=w707:errorcluster, "FP.State"=w705:T5)
            n335 = Not Equal?(x=w705, y=w703) -> (x != y?=w704:bool)
            n336 = case shown="True" w704 {
              tunnel: [w714 w715] -> w710
              tunnel: w707 -> [w713 w715]
              tunnel: w706 -> [w712 _]
              tunnel: w703 -> [w711 _]
              frame True {
                n337 = invoke class="VI" method="FP.Open"(reference=w712, error in=w713, "State"=w711) -> (error out=w714:errorcluster)  [unwired: 2 in, 4 out]
              }
              frame False {
              }
            }
          }
          frame "Minimize", "Minimized" {
            w716 = T5."Minimized" ("State")
            n338 = property class="VI"(reference=w722, error in=w721) -> (reference out=w719:refnum<vi>, error out=w720:errorcluster, "FP.State"=w718:T5)
            n339 = Not Equal?(x=w718, y=w716) -> (x != y?=w717:bool)
            n340 = case shown="True" w717 {
              tunnel: [w727 w728] -> w723
              tunnel: w720 -> [w726 w728]
              tunnel: w719 -> [w725 _]
              tunnel: w716 -> [w724 _]
              frame True {
                n341 = invoke class="VI" method="FP.Open"(reference=w725, error in=w726, "State"=w724) -> (error out=w727:errorcluster)  [unwired: 2 in, 4 out]
              }
              frame False {
              }
            }
          }
          frame "Maximize", "Maximized" {
            w729 = T5."Maximized" ("State")
            n342 = property class="VI"(reference=w735, error in=w734) -> (reference out=w732:refnum<vi>, error out=w733:errorcluster, "FP.State"=w731:T5)
            n343 = Not Equal?(x=w731, y=w729) -> (x != y?=w730:bool)
            n344 = case shown="True" w730 {
              tunnel: [w740 w741] -> w736
              tunnel: w733 -> [w739 w741]
              tunnel: w732 -> [w738 _]
              tunnel: w729 -> [w737 _]
              frame True {
                n345 = invoke class="VI" method="FP.Open"(reference=w738, error in=w739, "State"=w737) -> (error out=w740:errorcluster)  [unwired: 2 in, 4 out]
              }
              frame False {
              }
            }
          }
        }
        n346 = call <vilib>:"Add State(s) to Queue__jki_lib_state_machine.vi"("State(s) in (\"\")"=w676) -> ("States Out"=w675:string)  [unwired: 14 in]
      }
      frame "---------- Macro ----------" {
        # "Do not put any code in this frame.\n(It is a separator no-op. You can make a copy of this frame to create a new Macro frame)"
        n347 = call <vilib>:"Add State(s) to Queue__jki_lib_state_machine.vi"("State(s) in (\"\")"=w745) -> ("States Out"=w744:string)  [unwired: 14 in]
      }
      frame "Macro: Initialize" {
        # "Initialization Macro\n(This is called once, when the VI starts)"
        n348 = Unbundle By Name(w748) -> ("Run Time System?"=w747:bool)
        n349 = Select(t="", s=w747, f="Macro: Start Sweep") -> (s? t:f=w751:string)
        n350 = call <vilib>:"Add State(s) to Queue__jki_lib_state_machine.vi"("State(s) in Front (\"\")"="Data: Initialize\nInitialize Core Data\nUI: Initialize\nUI: Front Panel State >> Open\nData: Initialize Top Level\nMacro: Initialize Instruments", "State(s) at Back (\"\")"=w751) -> ("States Out"=w749:string)  [unwired: 13 in]
        n351 = call <vilib>:"Add State(s) to Queue__jki_lib_state_machine.vi"("State(s) in Front (\"\")"=w749, "State(s) in (\"\")"=w755) -> ("States Out"=w754:string)  [unwired: 13 in]
      }
      frame "Macro: Initialize Instruments" {
        # "Do not put any code in this frame.\n(It is a separator no-op. You can make a copy of this frame to create a new Macro frame)"
        n352 = call <vilib>:"Add State(s) to Queue__jki_lib_state_machine.vi"("State(s) in Front (\"\")"="Data: Initialize Instruments\nData: Disable Unsupported Instruments\nData: Open Instruments\nData: Configure Magnet Type" ("State(s) in Front (\"\")"), "State(s) in (\"\")"=w760) -> ("States Out"=w759:string)  [unwired: 13 in]
      }
      frame "Macro: Measure Instruments" {
        # "Do not put any code in this frame.\n(It is a separator no-op. You can make a copy of this frame to create a new Macro frame)"
        n353 = Unbundle By Name(w769) -> ("Instruments"=w768:T13)
        n354 = Cluster To Array(cluster=w768) -> (array=w767:refnum<class "Instrument.lvclass">[])
        n355 = for {
          tunnel: w767 -> [w778] mode=indexing
          tunnel: [w781] -> w765 mode=indexing if=w776
          tunnel: [w774] -> w763 mode=indexing
          n356 = call "Get IsConfigured.vi"("SMO"=w778) -> ("error out"=w775:errorcluster, "IsConfigured?"=w776:bool, "SMO out"=w777:refnum<class "Instrument.lvclass">)  [unwired: 8 in]
          n357 = call "Get StateName.vi"("error in (no error)"=w775, "SMO"=w777) -> ("error out"=w774:errorcluster, "StateName"=w779:string)  [unwired: 7 in, 1 out]
          n358 = Concatenate Strings("Measure: " ("string"), w779) -> (w781:string)
        }
        n359 = Merge Errors(w761, w763) -> (w762:errorcluster)
        n360 = call <vilib>:"1D String Array to Delimited String.vi"("delimiter"="\n", "string array"=w765) -> ("delimited string"=w764:string)  [unwired: 9 in]
        n361 = call <vilib>:"Add State(s) to Queue__jki_lib_state_machine.vi"("State(s) in Front (\"\")"="UI: Update Status >> reset" ("State(s) in Front (\"\")"), "State(s) at Back (\"\")"=w764) -> ("States Out"=w770:string)  [unwired: 13 in]
        n362 = call <vilib>:"Add State(s) to Queue__jki_lib_state_machine.vi"("State(s) in Front (\"\")"=w770, "State(s) in (\"\")"=w773) -> ("States Out"=w772:string)  [unwired: 13 in]
      }
      frame "Macro: Start Sweep" {
        # "Macro: Start Sweep\n()"
        n363 = call <vilib>:"Add State(s) to Queue__jki_lib_state_machine.vi"("State(s) in Front (\"\")"="Sweep: Initialize\nFile: Write JSON\nMeasure: Time\nMacro: Measure Instruments\nUI: Update AO AI Graphs >> reset\nUI: Update Lockin Graphs >> reset\nUI: Update R G Graphs\nUI: Update Lockin Graph Legend\nUI: Update Wfm Graph Legend\nUI: Update R G Graph Legend\nUI: Update Graph Axis Labels\nSweep: Start\nMeasure: DAQ\nUI: Update AO AI Graphs >> reset\nUI: Update Lockin Graphs >> reset\nUI: Update R G Graphs" ("State(s) in Front (\"\")"), "State(s) in (\"\")"=w786) -> ("States Out"=w785:string)  [unwired: 13 in]
      }
      frame "Macro: Sweep" {
        # "Template Separator\n(You can make a copy of, or modify, this frame)"
        n364 = call <vilib>:"Add State(s) to Queue__jki_lib_state_machine.vi"("State(s) in Front (\"\")"="Measure: Time\nMacro: Measure Instruments\nUI: Update AO AI Graphs\nUI: Update Lockin Graphs\nUI: Update R G Graphs\nUI: Update Timer" ("State(s) in Front (\"\")"), "State(s) in (\"\")"=w791) -> ("States Out"=w790:string)  [unwired: 13 in]
      }
      frame "Macro: Stop Sweep" {
        # "only \"return to start\"\nwhen stop button is pushed,\notherwise defer to sweep configuration"
        # "Macro: Stop Sweep\n(handle sweep finish: stop, save data, return to start)"
        n365 = Unbundle By Name(w795) -> ("UI stop"=w794:bool)
        n366 = local read "Return to Start"() -> (w792:bool)
        n367 = And(x=w794, y=w792) -> (x .and. y?=w793:bool)
        n368 = Select(t="", s=w793, f="//") -> (s? t:f=w798:string)
        n369 = Format Into String(format string="Sweep: Stop\nMeasure: DAQ Sweep\nUI: Update AO AI Graphs\nUI: Update IV Graphs\nUI: Update Graphs from wfm\nUI: Update R G Graphs\nFile: Save Lockin\n%sSweep: Return to Start" ("State(s) in Front (\"\")"), w798) -> (resulting string=w796:string)  [unwired: 2 in, 1 out]
        n370 = call <vilib>:"Add State(s) to Queue__jki_lib_state_machine.vi"("State(s) in Front (\"\")"=w796, "State(s) in (\"\")"=w803) -> ("States Out"=w802:string)  [unwired: 13 in]
      }
      frame "Macro: Exit" {
        # "Exit Macro\n(This is called once, when the VI exits)"
        n371 = Unbundle By Name(w811) -> ("Core.Close Panel on Exit?"=w810:bool)
        n372 = Select(t="UI: Front Panel State >> Close", s=w810, f="") -> (s? t:f=w807:string)
        n373 = call <vilib>:"Add State(s) to Queue__jki_lib_state_machine.vi"("State(s) in Front (\"\")"="Macro: Stop Sweep\nData: Close Instruments", "State(s) in (\"\")"=w807, "State(s) at Back (\"\")"="Data: Cleanup\nExit") -> ("States Out"=w806:string)  [unwired: 12 in]
        n374 = call <vilib>:"Add State(s) to Queue__jki_lib_state_machine.vi"("State(s) in Front (\"\")"=w806, "State(s) in (\"\")"=w814) -> ("States Out"=w813:string)  [unwired: 13 in]
      }
      frame "---------- Sweep ----------" {
        # "Do not put any code in this frame.\n(It is a separator no-op. You can make a copy of this frame to create a new Macro frame)"
        n375 = call <vilib>:"Add State(s) to Queue__jki_lib_state_machine.vi"("State(s) in (\"\")"=w818) -> ("States Out"=w817:string)  [unwired: 14 in]
      }
      frame "Sweep: Initialize" {
        # "If Running Top Level\nOR\nSweep Channels from Transport\nare empty, use FP controls"
        # "Do not put any code in this frame.\n(It is a separator no-op. You can make a copy of this frame to create a new Macro frame)"
        n376 = Unbundle By Name(w848) -> ("Instruments.DAQ"=w828:refnum<class "Instrument.LockinAPI.lvclass">, "Execution:State"=w835:T7, "Transport"=w832:refnum<class "Transport.lvclass">)
        n377 = Unbundle By Name(w832) -> ("sweepChannels"=w829:T2)
        n378 = Equal?(x=T7."Run top level" ("Execution:State"), y=w835) -> (x = y?=w833:bool)
        n379 = Empty Array?(array=w829) -> (empty?=w831:bool)
        n380 = Or(x=w833, y=w831) -> (x .or. y?=w830:bool)
        n381 = case shown="False" w830 {
          tunnel: "Sweep Time (s)" -> [_ w865]
          tunnel: [w858 w865] -> w838
          tunnel: "Initial Wait (s)" -> [_ w864]
          tunnel: [w859 w864] -> w839
          tunnel: [w856 w862] -> w840
          tunnel: "Sweep Channels" -> [_ w863]
          tunnel: [w857 w863] -> w841
          tunnel: w832 -> [w860 _]
          tunnel: "Sweep Tables" -> [_ w861]
          tunnel: "Return to Start" -> [_ w862]
          tunnel: [w855 w861] -> w836
          frame False {
            n382 = Unbundle By Name(w860) -> ("sweepTime"=w858:dbl, "initialWaitTime"=w859:dbl, "Return to Start"=w856:bool, "sweepChannels"=w857:T2, "sweepTables"=w855:cluster{"Ch":i32, "Table":dbl[]}[])
          }
          frame True {
          }
        }
        n383 = Bundle By Name(cluster=T10 {"sweepTime"=0.0, "initialWaitTime"=0.0, "returnToStart"=FALSE, "sweepChannels"=[]} ("Configure Sweep"), "sweepTime"=w838, "initialWaitTime"=w839, "returnToStart"=w840, "sweepChannels"=w841) -> (w846:T10)
        n384 = for {
          tunnel: [w853] -> w824 mode=indexing
          tunnel: [w852] -> w822 mode=indexing
          tunnel: w836 -> [w854] mode=indexing
          n385 = Unbundle By Name(w854) -> ("Ch"=w853:i32, "Table"=w852:dbl[])
        }
        n386 = local write "Sweep Time (s)"(w838) -> ()
        n387 = local write "Initial Wait (s)"(w839) -> ()
        n388 = local write "Return to Start"(w840) -> ()
        n389 = local write "Sweep Channels"(w841) -> ()
        n390 = local write "Sweep Tables"(w836) -> ()
        n391 = call "Cast Lockin tsc.vi"("error in (no error)"=w825, "Instrument.LockinAPI in"=w828) -> ("error out"=w826:errorcluster, "Instrument.Lockin out"=w827:refnum<class "Instrument.Lockin.lvclass">)  [unwired: 8 in]
        n392 = call-dynamic "setSweep.vi"("error in (no error)"=w826, "Configure Sweep"=w846, "Instrument.Lockin in"=w827) -> ("error out"=w820:errorcluster, "Instrument.Lockin out"=w823:refnum<class "Instrument.Lockin.lvclass">)  [unwired: 7 in]
        n393 = call "setSweepTable.vim"("error in (no error)"=w820, "Table"=w822, "Channel"=w824, "Instrument.Lockin in"=w823) -> ("error out"=w819:errorcluster, "Instrument.Lockin out"=w821:refnum<class "Instrument.Lockin.lvclass">)  [unwired: 6 in]
        n394 = Bundle By Name(cluster=w848, "Instruments.DAQ"=w821) -> (w849:T14)
        n395 = call <vilib>:"Add State(s) to Queue__jki_lib_state_machine.vi"("State(s) in (\"\")"=w851) -> ("States Out"=w850:string)  [unwired: 14 in]
      }
      frame "Sweep: Start" {
        # "wait for sweeping to start"
        # "Do not put any code in this frame.\n(It is a separator no-op. You can make a copy of this frame to create a new Macro frame)"
        n396 = Unbundle By Name(w875) -> ("Instruments.DAQ"=w869:refnum<class "Instrument.LockinAPI.lvclass">)
        n397 = call "Cast Lockin tsc.vi"("error in (no error)"=w866, "Instrument.LockinAPI in"=w869) -> ("error out"=w867:errorcluster, "Instrument.Lockin out"=w868:refnum<class "Instrument.Lockin.lvclass">)  [unwired: 8 in]
        n398 = call-dynamic "startSweep.vi"("error in (no error)"=w867, "Instrument.Lockin in"=w868) -> ("error out"=w873:errorcluster, "Instrument.Lockin out"=w872:refnum<class "Instrument.Lockin.lvclass">)  [unwired: 8 in]
        n399 = call-dynamic "waitStatusSweepingStarted.vi"("error in (no error)"=w873, "Instrument.Lockin in"=w872) -> ("error out"=w870:errorcluster, "Instrument.Lockin out"=w871:refnum<class "Instrument.Lockin.lvclass">)  [unwired: 8 in]
        n400 = Bundle By Name(cluster=w875, "Instruments.DAQ"=w871) -> (w874:T14)
        n401 = call <vilib>:"Add State(s) to Queue__jki_lib_state_machine.vi"("State(s) in (\"\")"=w877) -> ("States Out"=w876:string)  [unwired: 14 in]
      }
      frame "Sweep: Check State" {
        # "Sweep: Check State\n(It is a separator no-op. You can make a copy of this frame to create a new Macro frame)"
        n402 = Unbundle By Name(w883) -> ("Instruments.DAQ"=w881:refnum<class "Instrument.LockinAPI.lvclass">)
        n403 = call "Cast Lockin tsc.vi"("error in (no error)"=w878, "Instrument.LockinAPI in"=w881) -> ("error out"=w879:errorcluster, "Instrument.Lockin out"=w880:refnum<class "Instrument.Lockin.lvclass">)  [unwired: 8 in]
        n404 = call-dynamic "getStatus.vi"("error in (no error)"=w879, "Instrument.Lockin"=w880) -> ("error out"=w887:errorcluster, "state"=w886:T17, "Instrument.Lockin"=w882:refnum<class "Instrument.Lockin.lvclass">)  [unwired: 7 in]
        n405 = case shown="\"sweeping\"" w886 {
          tunnel: ["Macro: Exit" ("State(s) in Front (\"\")") "Macro: Sweep" ("State(s) in Front (\"\")")] -> w885
          frame Default {
          }
          frame "sweeping" {
          }
        }
        n406 = Bundle By Name(cluster=w883, "Instruments.DAQ"=w882) -> (w884:T14)
        n407 = call <vilib>:"Add State(s) to Queue__jki_lib_state_machine.vi"("State(s) in Front (\"\")"=w885, "State(s) in (\"\")"=w889) -> ("States Out"=w888:string)  [unwired: 13 in]
      }
      frame "Sweep: Stop" {
        # "Sweep: Stop\n(It is a separator no-op. You can make a copy of this frame to create a new Macro frame)"
        n408 = Unbundle By Name(w901) -> ("Instruments.DAQ"=w895:refnum<class "Instrument.LockinAPI.lvclass">)
        n409 = call "Cast Lockin tsc.vi"("error in (no error)"=w892, "Instrument.LockinAPI in"=w895) -> ("error out"=w893:errorcluster, "Instrument.Lockin out"=w894:refnum<class "Instrument.Lockin.lvclass">)  [unwired: 8 in]
        n410 = call-dynamic "stopSweep.vi"("error in (no error)"=w893, "Instrument.Lockin in"=w894) -> ("error out"=w899:errorcluster, "Instrument.Lockin out"=w898:refnum<class "Instrument.Lockin.lvclass">)  [unwired: 8 in]
        n411 = call-dynamic "waitStatusSweepingStopped.vi"("error in (no error)"=w899, "Instrument.Lockin in"=w898) -> ("error out"=w896:errorcluster, "Instrument.Lockin out"=w897:refnum<class "Instrument.Lockin.lvclass">)  [unwired: 8 in]
        n412 = Bundle By Name(cluster=w901, "Instruments.DAQ"=w897) -> (w900:T14)
        n413 = call <vilib>:"Add State(s) to Queue__jki_lib_state_machine.vi"("State(s) in (\"\")"=w903) -> ("States Out"=w902:string)  [unwired: 14 in]
      }
      frame "Sweep: Return to Start" {
        # "Sweep: Stop\n(It is a separator no-op. You can make a copy of this frame to create a new Macro frame)"
        n414 = local read "Sweep Channels"() -> (w923:T2)
        n415 = Unbundle By Name(w925) -> ("Instruments.DAQ"=w907:refnum<class "Instrument.LockinAPI.lvclass">)
        n416 = call "Cast Lockin tsc.vi"("error in (no error)"=w904, "Instrument.LockinAPI in"=w907) -> ("error out"=w905:errorcluster, "Instrument.Lockin out"=w906:refnum<class "Instrument.Lockin.lvclass">)  [unwired: 8 in]
        n417 = call-dynamic "getAOconfig.vi"("error in (no error)"=w905, "Instrument.Lockin in"=w906) -> ("error out"=w913:errorcluster, "AOconfig"=w922:T18, "Instrument.Lockin out"=w916:refnum<class "Instrument.Lockin.lvclass">)  [unwired: 7 in]
        n418 = for {
          tunnel: w923 -> [w933] mode=indexing
          tunnel: w922 -> [w935]
          tunnel: [w930] -> w917 mode=indexing
          n419 = Unbundle By Name(w933) -> ("Channel"=w932:u16, "Start"=w931:dbl)
          n420 = Decrement(x=w932) -> (x-1=w936:u16)
          n421 = Index Array(array=w935, index=w936) -> (element=w934:T19)
          n422 = Unbundle By Name(w934) -> ("Offset"=w929:dbl)
          n423 = Bundle By Name(cluster=w933, "Start"=w929, "End"=w931, "Pattern"=Sweep.Pattern--Enum."Smooth Ramp _/") -> (w930:T3)
        }
        n424 = Bundle By Name(cluster=T10 {"sweepTime"=0.0, "initialWaitTime"=0.0, "returnToStart"=FALSE, "sweepChannels"=[]} ("Configure Sweep"), "sweepTime"=2.0 ("Sweep Time (s)"), "sweepChannels"=w917) -> (w918:T10)
        n425 = call-dynamic "setSweep.vi"("error in (no error)"=w913, "Configure Sweep"=w918, "Instrument.Lockin in"=w916) -> ("error out"=w920:errorcluster, "Instrument.Lockin out"=w921:refnum<class "Instrument.Lockin.lvclass">)  [unwired: 7 in]
        n426 = call-dynamic "startSweep.vi"("error in (no error)"=w920, "Instrument.Lockin in"=w921) -> ("error out"=w912:errorcluster, "Instrument.Lockin out"=w911:refnum<class "Instrument.Lockin.lvclass">)  [unwired: 8 in]
        n427 = call-dynamic "waitStatusSweepingStarted.vi"("error in (no error)"=w912, "Instrument.Lockin in"=w911) -> ("error out"=w909:errorcluster, "Instrument.Lockin out"=w910:refnum<class "Instrument.Lockin.lvclass">)  [unwired: 8 in]
        n428 = call-dynamic "waitStatusSweepingStopped.vi"("error in (no error)"=w909, "Instrument.Lockin in"=w910) -> ("error out"=w914:errorcluster, "Instrument.Lockin out"=w915:refnum<class "Instrument.Lockin.lvclass">)  [unwired: 8 in]
        n429 = Bundle By Name(cluster=w925, "Instruments.DAQ"=w915) -> (w924:T14)
        n430 = call <vilib>:"Add State(s) to Queue__jki_lib_state_machine.vi"("State(s) in (\"\")"=w927) -> ("States Out"=w926:string)  [unwired: 14 in]
      }
      frame "---------- Configure ----------" {
        # "Do not put any code in this frame.\n(It is a separator no-op. You can make a copy of this frame to create a new Macro frame)"
        n431 = call <vilib>:"Add State(s) to Queue__jki_lib_state_machine.vi"("State(s) in (\"\")"=w940) -> ("States Out"=w939:string)  [unwired: 14 in]
      }
      frame "Configure: Wait" {
        # "Do not put any code in this frame.\n(It is a separator no-op. You can make a copy of this frame to create a new Macro frame)"
        n432 = call <vilib>:"Add State(s) to Queue__jki_lib_state_machine.vi"("State(s) in (\"\")"=w944) -> ("States Out"=w943:string)  [unwired: 14 in]
      }
      frame "---------- Measure ----------" {
        # "Template Separator\n(You can make a copy of, or modify, this frame)"
        n433 = call <vilib>:"Add State(s) to Queue__jki_lib_state_machine.vi"("State(s) in (\"\")"=w948) -> ("States Out"=w947:string)  [unwired: 14 in]
      }
      frame "Measure: Time" {
        # "Measure: Time.\n()"
        n434 = Unbundle By Name(w952) -> ("C.E."=w954:refnum<class "Control Experiment.lvclass">)
        n435 = Get Date/Time In Seconds() -> (seconds since 1Jan1904=w957:timestamp)
        n436 = To Double Precision Float(number=w957) -> (double precision float=w949:dbl)
        n437 = call "Write Dictionary Element.vi"("error in (no error)"=w951, "value"=w949, "key"="Time", "Control Experiment in"=w954) -> ("error out"=w950:errorcluster, "Control Experiment out"=w955:refnum<class "Control Experiment.lvclass">)  [unwired: 6 in]
        n438 = Bundle By Name(cluster=w952, "C.E."=w955, "Time"=w949) -> (w956:T14)
        n439 = call <vilib>:"Add State(s) to Queue__jki_lib_state_machine.vi"("State(s) in (\"\")"=w959) -> ("States Out"=w958:string)  [unwired: 14 in]
      }
      frame "Measure: Temperature" {
        # "Measure: Temperature.\n(called dynamically if instrument is configured in Control Experiment.vi)"
        n440 = Unbundle By Name(w968) -> ("Instruments.Temperature"=w966:refnum<class "Instrument.Cryostat.lvclass">, "C.E."=w970:refnum<class "Control Experiment.lvclass">)
        n441 = call-dynamic "getTemperature.vi"("error in (no error)"=w972, "Instrument.Cryostat in"=w966) -> ("error out"=w965:errorcluster, "Temperature (K)"=w961:dbl, "Instrument.Cryostat out"=w969:refnum<class "Instrument.Cryostat.lvclass">)  [unwired: 5 in, 2 out]
        n442 = call "Write Dictionary Element.vi"("error in (no error)"=w965, "value"=w961, "key"="Temperature", "Control Experiment in"=w970) -> ("error out"=w963:errorcluster, "Control Experiment out"=w967:refnum<class "Control Experiment.lvclass">)  [unwired: 6 in]
        n443 = case shown="No Error" w963 {
          selector: w963 -> [w975 w981]
          tunnel: w961 -> [w979 _]
          tunnel: [w976 _] -> w960
          tunnel: [w975 w981] -> w962
          frame No Error {
            n444 = Format Into String(format string="T = %2f K", w979) -> (resulting string=w977:string)  [unwired: 2 in, 1 out]
            n445 = call <vilib>:"Build State String with Arguments__JKI_lib_State_Machine.vi"("Arguments (\"\")"=w977, "State"="UI: Update Status" ("format string")) -> ("State with Arguments"=w976:string)  [unwired: 4 in]
          }
          frame Error {
          }
        }
        n446 = Bundle By Name(cluster=w968, "Instruments.Temperature"=w969, "C.E."=w967, "Temperature"=w961) -> (w971:T14)
        n447 = call <vilib>:"Add State(s) to Queue__jki_lib_state_machine.vi"("State(s) in Front (\"\")"=w960, "State(s) in (\"\")"=w974) -> ("States Out"=w973:string)  [unwired: 13 in]
      }
      frame "Measure: Magnet" {
        # "Measure: Magnet.\n(called dynamically by if instrument is configured in Control Experiment.vi)"
        n448 = Unbundle By Name(w989) -> ("Instruments.Magnet"=w988:refnum<class "Instrument.Cryostat.lvclass">, "C.E."=w992:refnum<class "Control Experiment.lvclass">)
        n449 = call-dynamic "getMagnet.vi"("error in (no error)"=w991, "Instrument.Cryostat in"=w988) -> ("error out"=w987:errorcluster, "B Field (T)"=w983:dbl, "Instrument.Cryostat out"=w990:refnum<class "Instrument.Cryostat.lvclass">)  [unwired: 5 in, 2 out]
        n450 = call "Write Dictionary Element.vi"("error in (no error)"=w987, "value"=w983, "key"="Magnet", "Control Experiment in"=w992) -> ("error out"=w985:errorcluster, "Control Experiment out"=w993:refnum<class "Control Experiment.lvclass">)  [unwired: 6 in]
        n451 = case shown="No Error" w985 {
          selector: w985 -> [w997 w1003]
          tunnel: w983 -> [w1001 _]
          tunnel: [w998 _] -> w982
          tunnel: [w997 w1003] -> w984
          frame No Error {
            n452 = Format Into String(format string="B = %2f T", w1001) -> (resulting string=w999:string)  [unwired: 2 in, 1 out]
            n453 = call <vilib>:"Build State String with Arguments__JKI_lib_State_Machine.vi"("Arguments (\"\")"=w999, "State"="UI: Update Status" ("format string")) -> ("State with Arguments"=w998:string)  [unwired: 4 in]
          }
          frame Error {
          }
        }
        n454 = Bundle By Name(cluster=w989, "Instruments.Magnet"=w990, "C.E."=w993, "Magnet"=w983) -> (w994:T14)
        n455 = call <vilib>:"Add State(s) to Queue__jki_lib_state_machine.vi"("State(s) in Front (\"\")"=w982, "State(s) in (\"\")"=w996) -> ("States Out"=w995:string)  [unwired: 13 in]
      }
      frame "Measure: Vector Magnet" {
        # "Measure: Vector Magnet.\n(called dynamically by if instrument is configured in Control Experiment.vi)"
        n456 = Unbundle By Name(w1015) -> ("Instruments.Magnet"=w1012:refnum<class "Instrument.Cryostat.lvclass">, "C.E."=w1022:refnum<class "Control Experiment.lvclass">)
        n457 = case shown="\"X\"" Magnet_Axis--Enum."Z" ("Axis") {
          tunnel: [2 ("index") 0 ("index") 1 ("index")] -> w1017
          frame "Z", Default {
          }
          frame "X" {
          }
          frame "Y" {
          }
        }
        n458 = call-dynamic "getMagnetVector.vi"("error in (no error)"=w1011, "Instrument.Cryostat in"=w1012) -> ("error out"=w1006:errorcluster, "Field (T)"=w1008:dbl[], "Instrument.Cryostat out"=w1010:refnum<class "Instrument.Cryostat.lvclass">)  [unwired: 5 in, 2 out]
        n459 = for {
          tunnel: w1008 -> [w1028] mode=indexing
          tunnel: string[] ["Bx", "By", "Bz"] ("input 1") -> [w1027] mode=indexing
          shift-right: [w1029] -> w1021
          shift-left: w1022 -> [w1030]
          tunnel: w1006 -> [w1026]
          tunnel: [w1025] -> w1007
          n460 = call "Write Dictionary Element.vi"("error in (no error)"=w1026, "value"=w1028, "key"=w1027, "Control Experiment in"=w1030) -> ("error out"=w1025:errorcluster, "Control Experiment out"=w1029:refnum<class "Control Experiment.lvclass">)  [unwired: 6 in]
        }
        n461 = Index Array(array=w1008, index #4=w1017) -> (element #1=w1020:dbl, element #2=w1019:dbl, element #3=w1018:dbl, element #4=w1009:dbl)  [unwired: 3 in]
        n462 = case shown="No Error" w1007 {
          selector: w1007 -> [w1036 w1042]
          tunnel: w1020 -> [w1040 _]
          tunnel: [w1037 _] -> w1004
          tunnel: [w1036 w1042] -> w1013
          tunnel: w1019 -> [w1035 _]
          tunnel: w1018 -> [w1034 _]
          frame No Error {
            n463 = Format Into String(format string="B = [%2f, %2f, %2f]", w1040, w1035, w1034) -> (resulting string=w1038:string)  [unwired: 2 in, 1 out]
            n464 = call <vilib>:"Build State String with Arguments__JKI_lib_State_Machine.vi"("Arguments (\"\")"=w1038, "State"="UI: Update Status" ("format string")) -> ("State with Arguments"=w1037:string)  [unwired: 4 in]
          }
          frame Error {
          }
        }
        n465 = Bundle By Name(cluster=w1015, "Instruments.Magnet"=w1010, "C.E."=w1021, "Magnet"=w1009) -> (w1016:T14)
        n466 = call <vilib>:"Add State(s) to Queue__jki_lib_state_machine.vi"("State(s) in Front (\"\")"=w1004, "State(s) in (\"\")"=w1024) -> ("States Out"=w1023:string)  [unwired: 13 in]
      }
      frame "Measure: Capacitance" {
        # "Measure: Capacitance.\n(called dynamically if instrument is configured in Control Experiment.vi)"
        n467 = Unbundle By Name(w1051) -> ("Instruments.Capacitance"=w1050:refnum<class "Instrument.CBridge.lvclass">, "C.E."=w1053:refnum<class "Control Experiment.lvclass">)
        n468 = call-dynamic "getCapacitance.vi"("error in (no error)"=w1052, "Instrument.CBridge in"=w1050) -> ("error out"=w1047:errorcluster, "Capacitance (pF)"=w1046:dbl, "Instrument.CBridge out"=w1049:refnum<class "Instrument.CBridge.lvclass">)  [unwired: 7 in]
        n469 = call "Write Dictionary Element.vi"("error in (no error)"=w1047, "value"=w1046, "key"="Capacitance", "Control Experiment in"=w1053) -> ("error out"=w1045:errorcluster, "Control Experiment out"=w1054:refnum<class "Control Experiment.lvclass">)  [unwired: 6 in]
        n470 = case shown="No Error" w1045 {
          selector: w1045 -> [w1058 w1064]
          tunnel: w1046 -> [w1062 _]
          tunnel: [w1059 _] -> w1043
          tunnel: [w1058 w1064] -> w1044
          frame No Error {
            n471 = Format Into String(format string="C = %2f pF", w1062) -> (resulting string=w1060:string)  [unwired: 2 in, 1 out]
            n472 = call <vilib>:"Build State String with Arguments__JKI_lib_State_Machine.vi"("Arguments (\"\")"=w1060, "State"="UI: Update Status" ("format string")) -> ("State with Arguments"=w1059:string)  [unwired: 4 in]
          }
          frame Error {
          }
        }
        n473 = Bundle By Name(cluster=w1051, "Instruments.Capacitance"=w1049, "C.E."=w1054) -> (w1055:T14)
        n474 = call <vilib>:"Add State(s) to Queue__jki_lib_state_machine.vi"("State(s) in Front (\"\")"=w1043, "State(s) in (\"\")"=w1057) -> ("States Out"=w1056:string)  [unwired: 13 in]
      }
      frame "Measure: Strain Cell" {
        # "Measure: Strain Cell.\n(called dynamically if instrument is configured in Control Experiment.vi)"
        n475 = Unbundle By Name(w1073) -> ("Instruments.Strain Cell"=w1072:refnum<class "Instrument.Strain.lvclass">, "C.E."=w1075:refnum<class "Control Experiment.lvclass">)
        n476 = call-dynamic "getStrain.vi"("error in (no error)"=w1074, "Instrument.Strain in"=w1072) -> ("error out"=w1069:errorcluster, "Strain (V)"=w1065:dbl, "Instrument.Strain out"=w1071:refnum<class "Instrument.Strain.lvclass">)  [unwired: 7 in]
        n477 = call "Write Dictionary Element.vi"("error in (no error)"=w1069, "value"=w1065, "key"="Strain", "Control Experiment in"=w1075) -> ("error out"=w1068:errorcluster, "Control Experiment out"=w1076:refnum<class "Control Experiment.lvclass">)  [unwired: 6 in]
        n478 = case shown="No Error" w1068 {
          selector: w1068 -> [w1080 w1086]
          tunnel: w1065 -> [w1084 _]
          tunnel: [w1081 _] -> w1066
          tunnel: [w1080 w1086] -> w1067
          frame No Error {
            n479 = Format Into String(format string="Strain = %2f V", w1084) -> (resulting string=w1082:string)  [unwired: 2 in, 1 out]
            n480 = call <vilib>:"Build State String with Arguments__JKI_lib_State_Machine.vi"("Arguments (\"\")"=w1082, "State"="UI: Update Status" ("format string")) -> ("State with Arguments"=w1081:string)  [unwired: 4 in]
          }
          frame Error {
          }
        }
        n481 = Bundle By Name(cluster=w1073, "Instruments.Strain Cell"=w1071, "C.E."=w1076) -> (w1077:T14)
        n482 = call <vilib>:"Add State(s) to Queue__jki_lib_state_machine.vi"("State(s) in Front (\"\")"=w1066, "State(s) in (\"\")"=w1079) -> ("States Out"=w1078:string)  [unwired: 13 in]
      }
      frame "Measure: Delay Line" {
        # "Measure: Delay Line.\n(called dynamically if instrument is configured in Control Experiment.vi)"
        n483 = Unbundle By Name(w1095) -> ("Instruments.Delay Line"=w1094:refnum<class "Instrument.DelayLine.lvclass">, "C.E."=w1097:refnum<class "Control Experiment.lvclass">)
        n484 = call-dynamic "getDelay.vi"("error in (no error)"=w1096, "Instrument.DelayLine in"=w1094) -> ("error out"=w1091:errorcluster, "delay (ps)"=w1087:dbl, "Instrument.DelayLine out"=w1093:refnum<class "Instrument.DelayLine.lvclass">)  [unwired: 6 in, 1 out]
        n485 = call "Write Dictionary Element.vi"("error in (no error)"=w1091, "value"=w1087, "key"="Delay", "Control Experiment in"=w1097) -> ("error out"=w1090:errorcluster, "Control Experiment out"=w1098:refnum<class "Control Experiment.lvclass">)  [unwired: 6 in]
        n486 = case shown="No Error" w1090 {
          selector: w1090 -> [w1102 w1108]
          tunnel: w1087 -> [w1106 _]
          tunnel: [w1103 _] -> w1088
          tunnel: [w1102 w1108] -> w1089
          frame No Error {
            n487 = Format Into String(format string="Delay = %2f ps", w1106) -> (resulting string=w1104:string)  [unwired: 2 in, 1 out]
            n488 = call <vilib>:"Build State String with Arguments__JKI_lib_State_Machine.vi"("Arguments (\"\")"=w1104, "State"="UI: Update Status" ("format string")) -> ("State with Arguments"=w1103:string)  [unwired: 4 in]
          }
          frame Error {
          }
        }
        n489 = Bundle By Name(cluster=w1095, "Instruments.Delay Line"=w1093, "C.E."=w1098) -> (w1099:T14)
        n490 = call <vilib>:"Add State(s) to Queue__jki_lib_state_machine.vi"("State(s) in Front (\"\")"=w1088, "State(s) in (\"\")"=w1101) -> ("States Out"=w1100:string)  [unwired: 13 in]
      }
      frame "Measure: Rotator" {
        # "Measure: Delay Line.\n(called dynamically if instrument is configured in Control Experiment.vi)"
        n491 = Unbundle By Name(w1117) -> ("Instruments.Rotator"=w1116:refnum<class "Instrument.Cryostat.lvclass">, "C.E."=w1119:refnum<class "Control Experiment.lvclass">)
        n492 = call-dynamic "getAngle.vi"("error in (no error)"=w1118, "Instrument.Cryostat in"=w1116) -> ("error out"=w1113:errorcluster, "Angle (°)"=w1109:dbl, "Instrument.Cryostat out"=w1115:refnum<class "Instrument.Cryostat.lvclass">)  [unwired: 5 in, 2 out]
        n493 = call "Write Dictionary Element.vi"("error in (no error)"=w1113, "value"=w1109, "key"="Angle", "Control Experiment in"=w1119) -> ("error out"=w1112:errorcluster, "Control Experiment out"=w1120:refnum<class "Control Experiment.lvclass">)  [unwired: 6 in]
        n494 = case shown="No Error" w1112 {
          selector: w1112 -> [w1124 w1130]
          tunnel: w1109 -> [w1128 _]
          tunnel: [w1125 _] -> w1110
          tunnel: [w1124 w1130] -> w1111
          frame No Error {
            n495 = Format Into String(format string="Angle = %2f°", w1128) -> (resulting string=w1126:string)  [unwired: 2 in, 1 out]
            n496 = call <vilib>:"Build State String with Arguments__JKI_lib_State_Machine.vi"("Arguments (\"\")"=w1126, "State"="UI: Update Status" ("format string")) -> ("State with Arguments"=w1125:string)  [unwired: 4 in]
          }
          frame Error {
          }
        }
        n497 = Bundle By Name(cluster=w1117, "Instruments.Rotator"=w1115, "C.E."=w1120) -> (w1121:T14)
        n498 = call <vilib>:"Add State(s) to Queue__jki_lib_state_machine.vi"("State(s) in Front (\"\")"=w1110, "State(s) in (\"\")"=w1123) -> ("States Out"=w1122:string)  [unwired: 13 in]
      }
      frame "Measure: DAQ" {
        # "Gives the AI and AO waveform which refreshes as per the Lockin sampling parameters"
        # "Measure Lockin\n(Read intermediate values of the waveforms)"
        n499 = Unbundle By Name(w1147) -> ("Instruments.DAQ"=w1134:refnum<class "Instrument.LockinAPI.lvclass">)
        n500 = local read "Sweep Channels"() -> (w1137:T2)
        n501 = call "Cast Lockin tsc.vi"("error in (no error)"=w1131, "Instrument.LockinAPI in"=w1134) -> ("error out"=w1132:errorcluster, "Instrument.Lockin out"=w1133:refnum<class "Instrument.Lockin.lvclass">)  [unwired: 8 in]
        n502 = for {
          tunnel: [w1156] -> w1136
          tunnel: w1137 -> [w1159] mode=indexing
          stop <- w1158 stop-if-true
          # "find the 1st enabled channel"
          n503 = Unbundle By Name(w1159) -> ("Enable?"=w1158:bool, "Channel"=w1157:u16)
          n504 = Decrement(x=w1157) -> (x-1=w1156:u16)
        }
        n505 = call-dynamic "getAOconfig.vi"("error in (no error)"=w1132, "Instrument.Lockin in"=w1133) -> ("error out"=w1139:errorcluster, "AOconfig"=w1135:T18, "Instrument.Lockin out"=w1142:refnum<class "Instrument.Lockin.lvclass">)  [unwired: 7 in]
        n506 = call-dynamic "getAOwfm.vi"("error in (no error)"=w1139, "Instrument.Lockin in"=w1142) -> ("error out"=w1149:errorcluster, "AO Waveforrm"=w1143:waveform(dbl)[], "Instrument.Lockin out"=w1151:refnum<class "Instrument.Lockin.lvclass">)  [unwired: 7 in]
        n507 = call-dynamic "getAIwfm.vi"("error in (no error)"=w1149, "Instrument.Lockin in"=w1151) -> ("error out"=w1148:errorcluster, "AI Waveform"=w1144:waveform(dbl)[], "Instrument.Lockin out"=w1150:refnum<class "Instrument.Lockin.lvclass">)  [unwired: 7 in]
        n508 = Index Array(array=w1135, index=w1136) -> (element=w1141:T19)
        n509 = for {
          tunnel: [w1161] -> w1138 mode=indexing
          tunnel: w1135 -> [w1160] mode=indexing
          n510 = Unbundle By Name(w1160) -> ("Amplitude"=w1161:dbl)
        }
        n511 = call-dynamic "getResults.vi"("error in (no error)"=w1148, "Instrument.Lockin in"=w1150) -> ("error out"=w1153:errorcluster, "Results (Dictionary)"=w1152:cluster{"key":string, "value":dbl}[], "Instrument.Lockin out"=w1145:refnum<class "Instrument.Lockin.lvclass">)  [unwired: 6 in, 1 out]
        n512 = Unbundle By Name(w1141) -> ("Offset"=w1140:dbl)
        n513 = Bundle By Name(cluster=w1147, "Instruments.DAQ"=w1145, "Results (Dictionary)"=w1152, "AI Waveform"=w1144, "AO Waveforrm"=w1143, "Amplitude"=w1138, "Sweep Value"=w1140) -> (w1146:T14)
        n514 = call <vilib>:"Add State(s) to Queue__jki_lib_state_machine.vi"("State(s) in (\"\")"=w1155) -> ("States Out"=w1154:string)  [unwired: 14 in]
      }
      frame "Measure: DAQ Sweep" {
        # "Gives the AI and AO waveform which refreshes as per the Lockin sampling parameters"
        # "Measure: Lockin Sweep\n(get all sweep waveforms from lockin)"
        n515 = Unbundle By Name(w1174) -> ("Instruments.DAQ"=w1165:refnum<class "Instrument.LockinAPI.lvclass">)
        n516 = call "Cast Lockin tsc.vi"("error in (no error)"=w1162, "Instrument.LockinAPI in"=w1165) -> ("error out"=w1163:errorcluster, "Instrument.Lockin out"=w1164:refnum<class "Instrument.Lockin.lvclass">)  [unwired: 8 in]
        n517 = call-dynamic "getSweepData.vi"("error in (no error)"=w1163, "Instrument.Lockin in"=w1164) -> ("error out"=w1171:errorcluster, "SweepData"=w1166:T21, "Instrument.Lockin out"=w1172:refnum<class "Instrument.Lockin.lvclass">)  [unwired: 7 in]
        n518 = Unbundle By Name(w1166) -> ("AO"=w1170:waveform(dbl)[], "AI"=w1169:waveform(dbl)[], "X"=w1168:waveform(dbl)[], "Y"=w1167:waveform(dbl)[])
        n519 = Bundle By Name(cluster=w1174, "Instruments.DAQ"=w1172, "Sweep_AO"=w1170, "Sweep_AI"=w1169, "Sweep_X"=w1168, "Sweep_Y"=w1167) -> (w1173:T14)
        n520 = call <vilib>:"Add State(s) to Queue__jki_lib_state_machine.vi"("State(s) in (\"\")"=w1176) -> ("States Out"=w1175:string)  [unwired: 14 in]
      }
      frame "---------- File ----------" {
        # "Template Separator\n(You can make a copy of, or modify, this frame)"
        n521 = call <vilib>:"Add State(s) to Queue__jki_lib_state_machine.vi"("State(s) in (\"\")"=w1180) -> ("States Out"=w1179:string)  [unwired: 14 in]
      }
      frame "File: Configure" {
        # "Template Separator\n(You can make a copy of, or modify, this frame)"
        n522 = call <vilib>:"Add State(s) to Queue__jki_lib_state_machine.vi"("State(s) in (\"\")"=w1184) -> ("States Out"=w1183:string)  [unwired: 14 in]
      }
      frame "File: Write JSON" {
        # "Template Separator\n(You can make a copy of, or modify, this frame)"
        n523 = Unbundle By Name(w1192) -> ("C.E."=w1190:refnum<class "Control Experiment.lvclass">)
        n524 = call "Write JSON to Dictionary.vi"("error in (no error)"=w1187, "Control Experiment in"=w1190) -> ("error out"=w1188:errorcluster, "Control Experiment out"=w1189:refnum<class "Control Experiment.lvclass">)  [unwired: 8 in]
        n525 = local read "Sweep Time (s)"() -> (w1199:dbl)
        n526 = local read "Initial Wait (s)"() -> (w1200:dbl)
        n527 = local read "Return to Start"() -> (w1201:bool)
        n528 = local read "Sweep Channels"() -> (w1202:T2)
        n529 = local read "Sweep Tables"() -> (w1185:cluster{"Ch":i32, "Table":dbl[]}[])
        n530 = Bundle By Name(cluster=T12 {"initialWaitTime"=0.0, "sweepTime"=0.0, "Return to Start"=FALSE, "sweepChannels"=[], "sweepTables"=[]} ("Lockin_Sweep"), "sweepTime"=w1199, "initialWaitTime"=w1200, "Return to Start"=w1201, "sweepChannels"=w1202, "sweepTables"=w1185) -> (w1197:T12)
        n531 = call "To JSON Text.vim"("error in (no error)"=w1188, "Anything"=w1197) -> ("error out"=w1191:errorcluster, "<JSON>"=w1198:string)  [unwired: 8 in]
        n532 = call "Write Dictionary Element.vi"("error in (no error)"=w1191, "value"=w1198, "key"="<LockinSweep>", "Control Experiment in"=w1189) -> ("error out"=w1195:errorcluster, "Control Experiment out"=w1194:refnum<class "Control Experiment.lvclass">)  [unwired: 6 in]
        n533 = Bundle By Name(cluster=w1192, "C.E."=w1194) -> (w1193:T14)
        n534 = call <vilib>:"Add State(s) to Queue__jki_lib_state_machine.vi"("State(s) in (\"\")"=w1204) -> ("States Out"=w1203:string)  [unwired: 14 in]
      }
      frame "File: Save Lockin" {
        # "F --> create\nnew file\neach time\nthis state runs"
        # "build cluster array(s) of multiple 1D data, dynamically name waves"
        # "Template Separator\n(You can make a copy of, or modify, this frame)"
        n535 = Unbundle By Name(w1218) -> ("C.E."=w1221:refnum<class "Control Experiment.lvclass">, "Sweep_AO"=w1210:waveform(dbl)[], "Sweep_AI"=w1209:waveform(dbl)[], "Sweep_X"=w1208:waveform(dbl)[], "Sweep_Y"=w1212:waveform(dbl)[])
        n536 = Build Cluster Array(w1210, w1209, w1208, w1212) -> (w1205:cluster{"Sweep_Y":waveform(dbl)[]}[])
        n537 = for {
          shift-right: [w1228] -> w1213
          shift-left: w1211 -> [w1229]
          tunnel: string[] ["AO", "AI", "X", "Y"] -> [w1227] mode=indexing
          tunnel: [w1226] -> w1206 mode=concatenating
          tunnel: w1205 -> [w1225] mode=indexing
          n538 = Unbundle(w1225) -> ("Sweep_Y"=w1224:waveform(dbl)[])
          n539 = call "Data to Dictionary.vim"("Error in"=w1229, "Data in"=w1224, "Label in"=w1227) -> ("Error out"=w1228:errorcluster, "Data out"=w1226:T22[])  [unwired: 7 in]
        }
        n540 = call "Write Dictionary Elements (Loop).vi"("error in (no error)"=w1213, "Data in"=w1206, "Control Experiment in"=w1221) -> ("error out"=w1215:errorcluster, "Control Experiment out"=w1217:refnum<class "Control Experiment.lvclass">)  [unwired: 7 in]
        n541 = call "Save Transport TDMS File.vi"("append?"=FALSE, "error in (no error)"=w1215, "Control Experiment in"=w1217) -> ("error out"=w1216:errorcluster, "Control Experiment out"=w1220:refnum<class "Control Experiment.lvclass">)  [unwired: 7 in]
        n542 = Bundle By Name(cluster=w1218, "C.E."=w1220) -> (w1219:T14)
        n543 = call <vilib>:"Add State(s) to Queue__jki_lib_state_machine.vi"("State(s) in (\"\")"=w1223) -> ("States Out"=w1222:string)  [unwired: 14 in]
      }
    }
  }
  "error out" <- w2
  n544 = Unbundle By Name(w4) -> ("Transport"=→"Transport out":refnum<class "Transport.lvclass">)
